vi "7.0.0_MAC Address reading.vi"(7 "Data in":T1, 8 "error in (no error)":errorcluster, 9 "AllControls In":T2, 10 "?":T3, 11 "Message Queue out":T4) -> (0 "error out":errorcluster, 1 "Flow":string, 2 "Data":T3, 3 "Message Queue Out":T4, 5 "Data out":T1)   [LabVIEW 2017]
uses:
  Depends/AMC/subVIs/TypeDefs/amc_Message Queue.ctl
  Depends/AMC/subVIs/TypeDefs/amc_Message.ctl
  Depends/Tools/Keyed Array/Tools_KeyedArray KeyedArray.ctl
  Ctrls/Data.ctl
  Ctrls/AllControls.ctl
  Ctrls/CSV_Data.ctl
  DIPC 692 Daemon API/typdef/destination.ctl
  DIPC 692 Daemon API/typdef/device_mode.ctl
  Ctrls/PathChoose.ctl
  DIPC 692 Daemon API/typdef/read_nvm_section.ctl
  DIPC 692 Daemon API/typdef/get_parameter.ctl
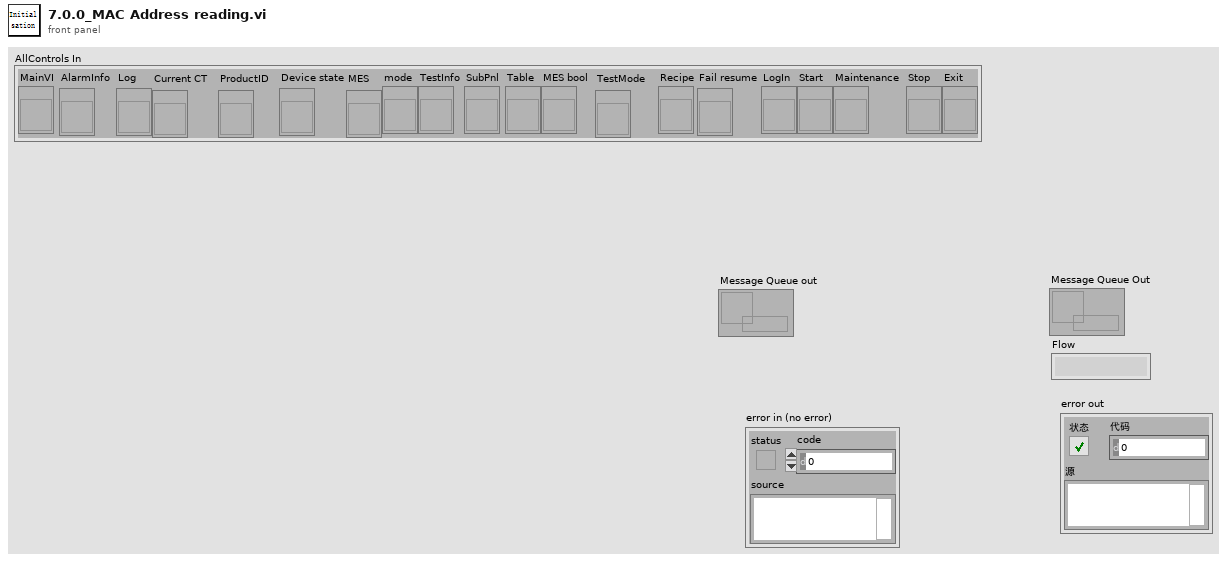
[diagram p1: front panel]
types:
  T1 = typedef "CSV_Data.ctl" = cluster{"Initialisation":cluster{"LMT - Connect UUT (con COM)":string, "LMT - Software Version (rrel)":string, "LMT - Write SKU file (wskuc)":string, "LMT - SKU file name":string, "Connect UUT DDM":string, "Read DDM EOL Timestamp - Mode":string, "Read DDM EOL Timestamp - Timestamp":string, "Read DDM EOL Timestamp - Rig ID":string, "Read DDM EOL Timestamp - Passmark ID":string, "Read DDM EOL Timestamp - Passmark Rev":string, "Software Version before flashing":string, "Read Hardware Serial":string, "UUT DDM SN":string, "Compare DDM SN with MES SN":string, "Backup PCBA Calibration EEPROM Response - CAL":string, "Flash Firmware Version":string, "Check SW Version":string, "Read DDM SW Version after flashing":string, "Set SKU Config":string, "Ready Status":string, "Set Device Mode to EOL":string, "DDM Parameter - Voltage":string, "DDM Parameter - Current":string, "DDM Parameter - Power":string, "DDM Parameter - Speed":string, "DDM Parameter - Pressure":string, "Tester Parameter - Voltage":string, "Tester Parameter - Current":string, "Tester Parameter - Power":string, "Tester Parameter - Ambient Pressure":string, "Tester Parameter - Ambient Temperature":string, "Calculated Parameter - DDM Pressure Corrected":string, "Calculated Parameter - DDM Real Power":string, "Calculated Parameter - Delta V":string}, "BEMF_Calibration":cluster{"Calibration Result - eol_cold_bemf_temp":string, "DDM Ambient Temp":string, "Restriction Plate Diameter":string, "Calibration Result - eol_bemf_mp_cold_coef_a":string, "Calibration Result - eol_bemf_mp_cold_coef_b":string, "Calibration Result - eol_bemf_mp_cold_coef_c":string, "Calibration Result - eol_bemf_lsi_cold_ref_coeffs":string, "Get - Calibration Result - eol_bemf_lsi_speed":string, "Get - Calibration Result - eol_bemf_lsi_integral_0":string, "Calibration Result - eol_bemf_lsi_integral_1":string, "Get - Calibration Result - eol_bemf_lsi_integral_2":string, "Get - Calibration Result - eol_cold_bemf":string, "Get - Calibration Result - eol_cold_bemf_fisf":string, "Finalise Calibration":string, "Compare -Calibration Result - eol_cold_bemf":string, "Compare -Calibration Result - eol_cold_bemf_fisf":string}, "ECO":cluster{"Reset Power Tune":string, "Reset BEMF FISF Calibration":string, "Restriction Plate Diameter":string, "ECO - Stabilisation Time":string, "ECO - DDM Parameter - Voltage":string, "ECO - DDM Parameter - Current":string, "ECO - DDM Parameter - Power":string, "ECO - DDM Parameter - Measured Power":string, "ECO - DDM Parameter - Speed":string, "ECO - DDM Parameter - Pressure":string, "ECO - Tester Parameter - Voltage":string, "ECO - Tester Parameter - Current":string, "ECO - Tester Parameter - Power":string, "ECO - Tester Parameter - Ambient Pressure":string, "ECO - Tester Parameter - Ambient Temperature":string, "ECO - Tester Parameter - Ambient Humidity":string, "ECO - Calculated Parameter - DDM Pressure Corrected":string, "ECO - Calculated Parameter - DDM Real Power":string, "ECO - Calculated Parameter - Delta V":string, "ECO - Calculated Parameter - Flowrate":string, "ECO - Calculated Parameter - Airwatt":string, "ECO - Formula":string, "PT ECO - Power Tune Mode Status":string}, "BOOST":cluster{"Restriction Plate Diameter":string, "BOOST - Stabilisation Time":string, "BOOST - DDM Parameter - Voltage":string, "BOOST - DDM Parameter - Current":string, "BOOST - DDM Parameter - Power":string, "BOOST - DDM Parameter - Measured Power":string, "BOOST - DDM Parameter - Speed":string, "BOOST - DDM Parameter - Pressure":string, "BOOST - Tester Parameter - Voltage":string, "BOOST - Tester Parameter - Current":string, "BOOST - Tester Parameter - Power":string, "BOOST - Tester Parameter - Ambient Pressure":string, "BOOST - Tester Parameter - Ambient Temperature":string, "BOOST - Tester Parameter - Ambient Humidity":string, "BOOST - Calculated Parameter - DDM Pressure Corrected":string, "BOOST - Calculated Parameter - DDM Real Power":string, "BOOST - Calculated Parameter - Delta V":string, "BOOST - Calculated Parameter - Flowrate":string, "BOOST - Calculated Parameter - Airwatt":string, "BOOST - Get AM Presence":string, "Air Muscle Turn Off Status":string, "BOOST - Air Muscle Calculated Parameter - Airwatt B":string, "BOOST - Air Muscle Calculate Airwatt Delta":string, "PT BOOST - Power Tune Mode Status":string, "Finalise Calibration":string, "ECO - Get AW Calibration value":string, "BOOST - Get AW Calibration value":string}, "MAX":cluster{"Restriction Plate Diameter":string, "MAX - Stabilisation Time":string, "Get Average Delta Tmag (LSIdelta_FISFdelta_LSItmag_FISFtmag_IIRtmag)":string, "Get Average Delta Tmag FISF":string, "MAX - DDM Parameter - Voltage":string, "MAX - DDM Parameter - Current":string, "MAX - DDM Parameter - Power":string, "MAX - DDM Parameter - Measured Power":string, "MAX - DDM Parameter - Speed":string, "MAX - DDM Parameter - Pressure":string, "MAX - Tester Parameter - Voltage":string, "MAX - Tester Parameter - Current":string, "MAX - Tester Parameter - Power":string, "MAX - Tester Parameter - Ambient Pressure":string, "MAX - Tester Parameter - Ambient Temperature":string, "MAX - Tester Parameter - Ambient Humidity":string, "MAX - Calculated Parameter - DDM Pressure Corrected":string, "MAX - Calculated Parameter - DDM Real Power":string, "MAX - Calculated Parameter - Delta V":string, "MAX - Calculated Parameter - Flowrate":string, "MAX - Calculated Parameter - Airwatt":string, "MAX_FISF_Check_Average_Delta_Tmag":string, "MAX - FISF - BEMF Finetune Result":string, "MAX tune - Delta P1":string, "MAX tune - Calculated Parameter - Airwatt":string, "Calculate Delta Airwatts - MAX finetune - Delta P2":string, "MAX finetune - DDM Parameter - Voltage":string, "MAX finetune - DDM Parameter - Current":string, "MAX finetune - DDM Parameter - Power":string, "MAX finetune - DDM Parameter - Measured Power":string, "MAX finetune - DDM Parameter - Speed":string, "MAX finetune - DDM Parameter - Pressure":string, "MAX finetune - Tester Parameter - Voltage":string, "MAX finetune - Tester Parameter - Current":string, "MAX finetune - Tester Parameter - Power":string, "MAX finetune - Tester Parameter - Ambient Pressure":string, "MAX finetune - Tester Parameter - Ambient Temperature":string, "MAX finetune - Tester Parameter - Ambient Humidity":string, "MAX finetune - Calculated Parameter - DDM Pressure Corrected":string, "MAX finetune - Calculated Parameter - DDM Real Power":string, "MAX finetune - Calculated Parameter - Delta V":string, "MAX finetune - Calculated Parameter - Flowrate":string, "MAX finetune - Calculated Parameter - Airwatt":string, "Check Derate Result":string, "Delta Tmag FISF":string, "Get Hot BEMF Result":string, "Calculate delta Pressure":string, "Finalise Calibration":string, "Calculate & Check Delta BEMF":string, "Delta P Airwatts Value":string}, "LL":cluster{"DDM Ambient Temp":string, "Restriction Plate Diameter":string, "LL - DDM Parameter - Voltage":string, "LL - DDM Parameter - Current":string, "LL - DDM Parameter - Power":string, "LL - DDM Parameter - Measured Power":string, "LL - DDM Parameter - Speed":string, "LL - DDM Parameter - Pressure":string, "LL - Tester Parameter - Voltage":string, "LL - Tester Parameter - Current":string, "LL - Tester Parameter - Power":string, "LL - DDM Real Power":string, "LL - Calibrate Task Detect LL":string}, "HL":cluster{"HL - DDM Parameter - Voltage":string, "HL - DDM Parameter - Current":string, "HL - DDM Parameter - Power":string, "HL - DDM Parameter - Measured Power":string, "HL - DDM Parameter - Speed":string, "HL - DDM Parameter - Pressure":string, "HL - Tester Parameter - Voltage":string, "HL - Tester Parameter - Current":string, "HL - Tester Parameter - Power":string, "HL - DDM Real Power":string, "HL - Calibrate Task Detect HL":string}, "LH":cluster{"Restriction Plate Diameter":string, "LH - DDM Parameter - Voltage":string, "LH - DDM Parameter - Current":string, "LH - DDM Parameter - Power":string, "LH - DDM Parameter - Measured Power":string, "LH - DDM Parameter - Speed":string, "LH - DDM Parameter - Pressure":string, "LH - Tester Parameter - Voltage":string, "LH - Tester Parameter - Current":string, "LH - Tester Parameter - Power":string, "LH - DDM Real Power":string, "LH - Calibrate Task Detect LH":string}, "HH":cluster{"HH - DDM Parameter - Voltage":string, "HH - DDM Parameter - Current":string, "HH - DDM Parameter - Power":string, "HH - DDM Parameter - Measured Power":string, "HH - DDM Parameter - Speed":string, "HH - DDM Parameter - Pressure":string, "HH - Tester Parameter - Voltage":string, "HH - Tester Parameter - Current":string, "HH - Tester Parameter - Power":string, "HH - DDM Real Power":string, "HH - Calibrate Task Detect HH":string}, "Inlet Blockage Calibration":cluster{"Inlet Blockage Calibration - DDM Parameter - Voltage":string, "Inlet Blockage Calibration - DDM Parameter - Current":string, "Inlet Blockage Calibration - DDM Parameter - Power":string, "Inlet Blockage Calibration - DDM Parameter - Measured Power":string, "Inlet Blockage Calibration - DDM Parameter - Speed":string, "Inlet Blockage Calibration - DDM Parameter - Pressure":string, "Inlet Blockage Calibration - Tester Parameter - Voltage":string, "Inlet Blockage Calibration - Tester Parameter - Current":string, "Inlet Blockage Calibration - Tester Parameter - Power":string, "Inlet Blockage Calibration - DDM Real Power":string, "Calibration Inlet Blockage_E":string, "Finalise Calibration":string, "Get Task Detect LL":string, "Get Task Detect HL":string, "Get Task Detect LH":string, "Get Task Detect HH":string, "Calibration Inlet Blockage":string, "Calibration eol cold bemf temp":string}, "GOOD":cluster{"GOOD UNIT - Clear EEPROM Error Log":string, "GOOD UNIT - Write Product Timestamp - Mode":string, "GOOD UNIT - Write Product Timestamp - Timestamp":string, "GOOD UNIT - Write Product Timestamp - Rig ID":string, "GOOD UNIT - Write Product Timestamp - Passmark ID":string, "GOOD UNIT - Write Product Timestamp - Passmark Rev":string, "GOOD UNIT - Set Device Mode to PROD":string, "GOOD UNIT - Backup PCBA Calibration EEPROM Response":string, "GOOD UNIT - Check Security Bit":string, "GOOD UNIT - Set Calibration Lock":string, "GOOD UNIT - Get_Calibration_Lock":string, "GOOD UNIT - Disconnect UUT":string}, "NG":cluster{"NG UNIT - Read NVM Error":string, "NG UNIT - Set Device Mode to FCT":string, "NG UNIT - Backup PCBA Calibration EEPROM Response - CAL":string, "NG UNIT - Backup PCBA Calibration EEPROM Response - ERROR":string, "NG UNIT - Backup PCBA Calibration EEPROM Response - USAGE":string, "NG UNIT - Disconnect UUT":string}, "SN":string, "Table":string[][], "Count":cluster{"Total":i32, "OK":i32, "NG":i32, "Yield":dbl}, "Start Time":timestamp, "daemon reference":refnum<k5>, "CT":dbl, "Config":string[][], "OK/NG":bool, "Station ID":string, "MES DDM SN":string, "MES PCBA SN":string, "Retest":string, "Lux":string, "Initialisation_Status":cluster{"LMT - Connect UUT (con COM)":string, "LMT - Software Version (rrel)":string, "LMT - Write SKU file (wskuc)":string, "LMT - SKU file name":string, "Connect UUT DDM":string, "Read DDM EOL Timestamp - Mode":string, "Read DDM EOL Timestamp - Timestamp":string, "Read DDM EOL Timestamp - Rig ID":string, "Read DDM EOL Timestamp - Passmark ID":string, "Read DDM EOL Timestamp - Passmark Rev":string, "Software Version before flashing":string, "Read Hardware Serial":string, "UUT DDM SN":string, "Compare DDM SN with MES SN":string, "Backup PCBA Calibration EEPROM Response - CAL":string, "Flash Firmware Version":string, "Check SW Version":string, "Read DDM SW Version after flashing":string, "Set SKU Config":string, "Ready Status":string, "Set Device Mode to EOL":string, "DDM Parameter - Voltage":string, "DDM Parameter - Current":string, "DDM Parameter - Power":string, "DDM Parameter - Speed":string, "DDM Parameter - Pressure":string, "Tester Parameter - Voltage":string, "Tester Parameter - Current":string, "Tester Parameter - Power":string, "Tester Parameter - Ambient Pressure":string, "Tester Parameter - Ambient Temperature":string, "Calculated Parameter - DDM Pressure Corrected":string, "Calculated Parameter - DDM Real Power":string, "Calculated Parameter - Delta V":string}, "BEMF_Calibration_Status":cluster{"Calibration Result - eol_cold_bemf_temp":string, "DDM Ambient Temp":string, "Restriction Plate Diameter":string, "Calibration Result - eol_bemf_mp_cold_coef_a":string, "Calibration Result - eol_bemf_mp_cold_coef_b":string, "Calibration Result - eol_bemf_mp_cold_coef_c":string, "Calibration Result - eol_bemf_lsi_cold_ref_coeffs":string, "Get - Calibration Result - eol_bemf_lsi_speed":string, "Get - Calibration Result - eol_bemf_lsi_integral_0":string, "Calibration Result - eol_bemf_lsi_integral_1":string, "Get - Calibration Result - eol_bemf_lsi_integral_2":string, "Get - Calibration Result - eol_cold_bemf":string, "Get - Calibration Result - eol_cold_bemf_fisf":string, "Finalise Calibration":string, "Compare -Calibration Result - eol_cold_bemf":string, "Compare -Calibration Result - eol_cold_bemf_fisf":string}, "ECO_Status":cluster{"Reset Power Tune":string, "Reset BEMF FISF Calibration":string, "Restriction Plate Diameter":string, "ECO - Stabilisation Time":string, "ECO - DDM Parameter - Voltage":string, "ECO - DDM Parameter - Current":string, "ECO - DDM Parameter - Power":string, "ECO - DDM Parameter - Measured Power":string, "ECO - DDM Parameter - Speed":string, "ECO - DDM Parameter - Pressure":string, "ECO - Tester Parameter - Voltage":string, "ECO - Tester Parameter - Current":string, "ECO - Tester Parameter - Power":string, "ECO - Tester Parameter - Ambient Pressure":string, "ECO - Tester Parameter - Ambient Temperature":string, "ECO - Tester Parameter - Ambient Humidity":string, "ECO - Calculated Parameter - DDM Pressure Corrected":string, "ECO - Calculated Parameter - DDM Real Power":string, "ECO - Calculated Parameter - Delta V":string, "ECO - Calculated Parameter - Flowrate":string, "ECO - Calculated Parameter - Airwatt":string, "ECO - Formula":string, "PT ECO - Power Tune Mode Status":string}, "BOOST_Status":cluster{"Restriction Plate Diameter":string, "BOOST - Stabilisation Time":string, "BOOST - DDM Parameter - Voltage":string, "BOOST - DDM Parameter - Current":string, "BOOST - DDM Parameter - Power":string, "BOOST - DDM Parameter - Measured Power":string, "BOOST - DDM Parameter - Speed":string, "BOOST - DDM Parameter - Pressure":string, "BOOST - Tester Parameter - Voltage":string, "BOOST - Tester Parameter - Current":string, "BOOST - Tester Parameter - Power":string, "BOOST - Tester Parameter - Ambient Pressure":string, "BOOST - Tester Parameter - Ambient Temperature":string, "BOOST - Tester Parameter - Ambient Humidity":string, "BOOST - Calculated Parameter - DDM Pressure Corrected":string, "BOOST - Calculated Parameter - DDM Real Power":string, "BOOST - Calculated Parameter - Delta V":string, "BOOST - Calculated Parameter - Flowrate":string, "BOOST - Calculated Parameter - Airwatt":string, "BOOST - Get AM Presence":string, "Air Muscle Turn Off Status":string, "BOOST - Air Muscle Calculated Parameter - Airwatt B":string, "BOOST - Air Muscle Calculate Airwatt Delta":string, "PT BOOST - Power Tune Mode Status":string, "Finalise Calibration":string, "ECO - Get AW Calibration value":string, "BOOST - Get AW Calibration value":string}, "MAX_Status":cluster{"Restriction Plate Diameter":string, "MAX - Stabilisation Time":string, "Get Average Delta Tmag (LSIdelta_FISFdelta_LSItmag_FISFtmag_IIRtmag)":string, "Get Average Delta Tmag FISF":string, "MAX - DDM Parameter - Voltage":string, "MAX - DDM Parameter - Current":string, "MAX - DDM Parameter - Power":string, "MAX - DDM Parameter - Measured Power":string, "MAX - DDM Parameter - Speed":string, "MAX - DDM Parameter - Pressure":string, "MAX - Tester Parameter - Voltage":string, "MAX - Tester Parameter - Current":string, "MAX - Tester Parameter - Power":string, "MAX - Tester Parameter - Ambient Pressure":string, "MAX - Tester Parameter - Ambient Temperature":string, "MAX - Tester Parameter - Ambient Humidity":string, "MAX - Calculated Parameter - DDM Pressure Corrected":string, "MAX - Calculated Parameter - DDM Real Power":string, "MAX - Calculated Parameter - Delta V":string, "MAX - Calculated Parameter - Flowrate":string, "MAX - Calculated Parameter - Airwatt":string, "MAX_FISF_Check_Average_Delta_Tmag":string, "MAX - FISF - BEMF Finetune Result":string, "MAX tune - Delta P1":string, "MAX tune - Calculated Parameter - Airwatt":string, "Calculate Delta Airwatts - MAX finetune - Delta P2":string, "MAX finetune - DDM Parameter - Voltage":string, "MAX finetune - DDM Parameter - Current":string, "MAX finetune - DDM Parameter - Power":string, "MAX finetune - DDM Parameter - Measured Power":string, "MAX finetune - DDM Parameter - Speed":string, "MAX finetune - DDM Parameter - Pressure":string, "MAX finetune - Tester Parameter - Voltage":string, "MAX finetune - Tester Parameter - Current":string, "MAX finetune - Tester Parameter - Power":string, "MAX finetune - Tester Parameter - Ambient Pressure":string, "MAX finetune - Tester Parameter - Ambient Temperature":string, "MAX finetune - Tester Parameter - Ambient Humidity":string, "MAX finetune - Calculated Parameter - DDM Pressure Corrected":string, "MAX finetune - Calculated Parameter - DDM Real Power":string, "MAX finetune - Calculated Parameter - Delta V":string, "MAX finetune - Calculated Parameter - Flowrate":string, "MAX finetune - Calculated Parameter - Airwatt":string, "Check Derate Result":string, "Delta Tmag FISF":string, "Get Hot BEMF Result":string, "Calculate delta Pressure":string, "Finalise Calibration":string, "Calculate & Check Delta BEMF":string, "Delta P Airwatts Value":string}, "LL_Status":cluster{"DDM Ambient Temp":string, "Restriction Plate Diameter":string, "LL - DDM Parameter - Voltage":string, "LL - DDM Parameter - Current":string, "LL - DDM Parameter - Power":string, "LL - DDM Parameter - Measured Power":string, "LL - DDM Parameter - Speed":string, "LL - DDM Parameter - Pressure":string, "LL - Tester Parameter - Voltage":string, "LL - Tester Parameter - Current":string, "LL - Tester Parameter - Power":string, "LL - DDM Real Power":string, "LL - Calibrate Task Detect LL":string}, "HL_Status":cluster{"HL - DDM Parameter - Voltage":string, "HL - DDM Parameter - Current":string, "HL - DDM Parameter - Power":string, "HL - DDM Parameter - Measured Power":string, "HL - DDM Parameter - Speed":string, "HL - DDM Parameter - Pressure":string, "HL - Tester Parameter - Voltage":string, "HL - Tester Parameter - Current":string, "HL - Tester Parameter - Power":string, "HL - DDM Real Power":string, "HL - Calibrate Task Detect HL":string}, "LH_Status":cluster{"Restriction Plate Diameter":string, "LH - DDM Parameter - Voltage":string, "LH - DDM Parameter - Current":string, "LH - DDM Parameter - Power":string, "LH - DDM Parameter - Measured Power":string, "LH - DDM Parameter - Speed":string, "LH - DDM Parameter - Pressure":string, "LH - Tester Parameter - Voltage":string, "LH - Tester Parameter - Current":string, "LH - Tester Parameter - Power":string, "LH - DDM Real Power":string, "LH - Calibrate Task Detect LH":string}, "HH_Status":cluster{"HH - DDM Parameter - Voltage":string, "HH - DDM Parameter - Current":string, "HH - DDM Parameter - Power":string, "HH - DDM Parameter - Measured Power":string, "HH - DDM Parameter - Speed":string, "HH - DDM Parameter - Pressure":string, "HH - Tester Parameter - Voltage":string, "HH - Tester Parameter - Current":string, "HH - Tester Parameter - Power":string, "HH - DDM Real Power":string, "HH - Calibrate Task Detect HH":string}, "Inlet Blockage Calibration_Status":cluster{"Inlet Blockage Calibration - DDM Parameter - Voltage":string, "Inlet Blockage Calibration - DDM Parameter - Current":string, "Inlet Blockage Calibration - DDM Parameter - Power":string, "Inlet Blockage Calibration - DDM Parameter - Measured Power":string, "Inlet Blockage Calibration - DDM Parameter - Speed":string, "Inlet Blockage Calibration - DDM Parameter - Pressure":string, "Inlet Blockage Calibration - Tester Parameter - Voltage":string, "Inlet Blockage Calibration - Tester Parameter - Current":string, "Inlet Blockage Calibration - Tester Parameter - Power":string, "Inlet Blockage Calibration - DDM Real Power":string, "Calibration Inlet Blockage_E":string, "Finalise Calibration":string, "Get Task Detect LL":string, "Get Task Detect HL":string, "Get Task Detect LH":string, "Get Task Detect HH":string, "Calibration Inlet Blockage":string, "Calibration eol cold bemf temp":string}, "GOOD_Status":cluster{"GOOD UNIT - Clear EEPROM Error Log":string, "GOOD UNIT - Write Product Timestamp - Mode":string, "GOOD UNIT - Write Product Timestamp - Timestamp":string, "GOOD UNIT - Write Product Timestamp - Rig ID":string, "GOOD UNIT - Write Product Timestamp - Passmark ID":string, "GOOD UNIT - Write Product Timestamp - Passmark Rev":string, "GOOD UNIT - Set Device Mode to PROD":string, "GOOD UNIT - Backup PCBA Calibration EEPROM Response":string, "GOOD UNIT - Check Security Bit":string, "GOOD UNIT - Set Calibration Lock":string, "GOOD UNIT - Get_Calibration_Lock":string, "GOOD UNIT - Disconnect UUT":string}, "NG_Status":cluster{"NG UNIT - Read NVM Error":string, "NG UNIT - Set Device Mode to FCT":string, "NG UNIT - Backup PCBA Calibration EEPROM Response - CAL":string, "NG UNIT - Backup PCBA Calibration EEPROM Response - ERROR":string, "NG UNIT - Backup PCBA Calibration EEPROM Response - USAGE":string, "NG UNIT - Disconnect UUT":string}, "SKU":string, "Plate_Diameter":string, "Alarm":string}
  T2 = typedef "AllControls.ctl" = cluster{"MainVI":refnum<vi>, "AlarmInfo":refnum<vi>, "Log":refnum<vi>, "Current CT":refnum<vi>, "ProductID":refnum<vi>, "Device state":refnum<vi>, "MES":refnum<vi>, "mode":refnum<vi>, "TestInfo":refnum<vi>, "SubPnl":refnum<vi>, "Table":refnum<vi>, "MES bool":refnum<vi>, "TestMode":refnum<vi>, "Recipe":refnum<vi>, "Fail resume":refnum<vi>, "LogIn":refnum<vi>, "Start":refnum<vi>, "Maintenance":refnum<vi>, "Stop":refnum<vi>, "Exit":refnum<vi>}
  T3 = typedef "Data.ctl" = cluster{"Initialisation":cluster{"DDM_Parameter":dbl[], "DDM_Parameter_status":bool[], "Get_Tester_Parameter":dbl[], "Get_Tester_Parameter_status":bool[], "Cal_Tester_Parameter":dbl[], "Cal_Tester_Parameter_status":bool[], "sw_version_before_status":bool, "sw_version_after_status":bool, "Set_SKU_Config_With_LMT_status":bool, "FCT_timestamp_status":bool, "LMT_Connect_to_UUT_status":bool}, "BEMF_Calibration":cluster{"Read_ambient_temperature":dbl, "Calibration_Vaule":dbl[], "Calibration_Vaule _B":dbl[], "Calibration_Vaule_status":bool[], "Calibration_Vaule_B_status":bool[]}, "ECO":cluster{"DDM_Parameter":dbl[], "DDM_Parameter_status":bool[], "Get_Tester_Parameter":dbl[], "Get_Tester_Parameter_status":bool[], "Cal_Tester_Parameter":dbl[], "Cal_Tester_Parameter_status":bool[], "DDM_Parameter_after_power_tune":dbl[], "Get_Tester_Parameter_after_power_tune":dbl[], "Cal_Tester_Parameter_after_power_tune":dbl[], "Cal_Tester_Parameter_after_power_tune_status":bool[], "Delta_P":dbl}, "BOOST":cluster{"DDM_Parameter":dbl[], "DDM_Parameter_status":bool[], "Get_Tester_Parameter":dbl[], "Get_Tester_Parameter_status":bool[], "Cal_Tester_Parameter":dbl[], "Cal_Tester_Parameter_status":bool[], "DDM_Parameter_after_power_tune":dbl[], "Get_Tester_Parameter_after_power_tune":dbl[], "Cal_Tester_Parameter_after_power_tune":dbl[], "Cal_Tester_Parameter_after_power_tune_status":bool[], "airwatts_am_off":dbl, "AW_Delta_(AM_on_and_off)":dbl, "AW_Delta_(AM_on_and_off)_Status":bool, "Delta_P":dbl}, "MAX":cluster{"Average_Tmag_Data":cluster{"LSI Delta in degC":dbl, "FISF Delta in degc":dbl, "LSI Tmag in degC":dbl, "Fisf Tmag in degC":dbl, "IIR Tmag in degC":dbl}, "DDM_Parameter":dbl[], "DDM_Parameter_status":bool[], "Get_Tester_Parameter":dbl[], "Get_Tester_Parameter_status":bool[], "Cal_Tester_Parameter":dbl[], "BEMF_Finetune":cluster{"eol_bemf_mp_cold_coef_c":dbl, "eol_cold_bemf_fisf_offset":dbl}, "AW_Tune":cluster{"delta_P1":dbl, "delta_P_Setting":dbl}, "DDM_Parameter_after_Airwatts_Tune":dbl[], "Get_Tester_Parameter_after_Airwatts_Tune":dbl[], "Cal_Tester_Parameter_after_Airwatts_Tune":dbl[], "DDM_Parameter_after_Airwatts_Finetune":dbl[], "Get_Tester_Parameter_after_Airwatts_Finetune":dbl[], "Cal_Tester_Parameter_after_Airwatts_Finetune":dbl[], "AW_Finetune":cluster{"delta_P2":dbl, "delta_P_Setting":dbl}, "Delta_Tmag_after_tune":cluster{"LSI Delta in degC":dbl, "FISF Delta in degc":dbl, "LSI Tmag in degC":dbl, "Fisf Tmag in degC":dbl, "IIR Tmag in degC":dbl}, "Hot Bemf in mV":dbl, "DDM_Pressure":dbl, "Delta_Pressure":dbl, " Cold Bemf in mV":dbl, " delta Bemf":dbl, " delta p":dbl, "Delta_Pressure_status":bool, " delta Bemf_status":bool, "LSI Delta in degC_status":bool, "FISF Delta in degc_status":bool, "Max_check_derate_status_status":bool, "Average_All_data":dbl[][], "Average_Tmag_Data_status":bool[], "Average_Tmag_Data_after_tune_status":bool[], "Cal_Tester_Parameter_status":bool[], "Cal_Tester_Parameter_status_after_Airwatts_Tune":bool[], "Cal_Tester_Parameter_status_after_Airwatts_FineTune":bool[]}, "Task_Detect_Calib":cluster{"LL":cluster{"DDM_Parameter":dbl[], "DDM_Parameter_status":bool[], "Get_Tester_Parameter":dbl[], "Get_Tester_Parameter_status":bool[], "Set_task_detect_A":dbl, "Set_task_detect_A_Status":bool}, "HL":cluster{"DDM_Parameter":dbl[], "DDM_Parameter_status":bool[], "Get_Tester_Parameter":dbl[], "Get_Tester_Parameter_status":bool[], "Set_task_detect_B":dbl, "Set_task_detect_B_Status":bool}, "LH":cluster{"DDM_Parameter":dbl[], "DDM_Parameter_status":bool[], "Get_Tester_Parameter":dbl[], "Get_Tester_Parameter_status":bool[], "Set_task_detect_C":dbl, "Set_task_detect_C_Status":bool}, "HH":cluster{"DDM_Parameter":dbl[], "DDM_Parameter_status":bool[], "Get_Tester_Parameter":dbl[], "Get_Tester_Parameter_status":bool[], "Set_task_detect_D":dbl, "Read_and_check_calibration_Status":bool[], "Set_task_detect_D_Status":bool}, "Get_eol_inlet_blockage_E":dbl, "Calib_vaule":cluster{"Get_task_detect_LL":dbl, "Get_task_detect_HL":dbl, "Get_task_detect_LH":dbl, "Get_task_detect_HH":dbl, "eol_inlet_blockage":dbl, "eol_code_bemf_temp":dbl}, "calibrated temp":dbl, "Inlet_Blockage_Calibration":cluster{"DDM_Parameter":dbl[], "DDM_Parameter_status":bool[], "Get_Tester_Parameter":dbl[], "Get_Tester_Parameter_status":bool[]}, "Get_eol_inlet_blockage_E_Status":bool}, "good":cluster{"Write_Product_TS":cluster{"TIMESTAMP":i64, "RIG_ID":i64, "PASSMARK_ID":i64, "PASSMARK_REV":i64}, "Read_Product_TS":cluster{"TIMESTAMP":i64, "RIG_ID":i64, "PASSMARK_ID":i64, "PASSMARK_REV":i64}, "Good_Check_Secuity_Bit_Stauts":bool}}
  T4 = typedef "amc_Message Queue.ctl" = refnum<queue>
  T5 = cluster{"Brush_ADC.bat":string, "Get Release Version.bat":string, "Getting Software  Version.bat":string, "Pump_ADC.bat":string, "Starting  Pump Motor.bat":string, "Starting  Test Mode.bat":string, "Starting Brush Motor 1.bat":string, "Starting Brush Motor 2.bat":string, "Starting Brush Motor 3.bat":string, "Starting LED Test.bat":string, "Stopping  Brush Motor.bat":string, "Stopping  Pump Motor.bat":string, "Stopping  Test Mode.bat":string, "1":string, "2":string, "3":string, "4":string, "5":string, "6":string, "7":string, "8":string, "9":string, "10":string}
  T6 = typedef "destination.ctl" = string
  T7 = typedef "PathChoose.ctl" = enum16{"OperatorLog", "AutoRunLog", "AlmLog", "TestData", "AllTestData", "backup_nvm", "backup_before_flashing"}
  T8 = enum16{"open", "replace", "create", "open or create", "replace or create", "replace or create with confirmation"}
  T9 = typedef "read_nvm_section.ctl" = enum16{"CAL", "ERROR", "USAGE"}
  T10 = typedef "get_parameter.ctl" = string
  T11 = typedef "HD Config.ctl" = cluster{" PC":cluster{"PC Address":u8[], "PC Port":i32}, "FCO":cluster{"COM":refnum<visa-resource-name>, "Baudrate":u32}, "DC Power ":cluster{"COM":refnum<visa-resource-name>, "Baudrate":u32}, "PW3336":cluster{"COM":refnum<visa-resource-name>, "Baudrate":u32}, "Lefoo":cluster{"COM":refnum<visa-resource-name>, "Baudrate":u32}, "Tempt&Hum":cluster{"COM":refnum<visa-resource-name>, "Baudrate":u32}, "DIPC":cluster{"COM":refnum<visa-resource-name>}, "Daemon":cluster{"IP Address":string, "Port":u16, "Retry":u16}, "URAT":cluster{"COM":refnum<visa-resource-name>, "Baudrate":u32}, "Fail_resume_mode":bool, "GRR":bool}
  T12 = typedef "device_mode.ctl" = enum16{"FCT", "EOL", "PROD"}
  T13 = cluster{"TIMESTAMP":i64, "RIG_ID":i64, "PASSMARK_ID":i64, "PASSMARK_REV":i64}
  T14 = cluster{"TIMESTAMP":string, "RIG_ID":string, "PASSMARK_ID":string, "PASSMARK_REV":string}
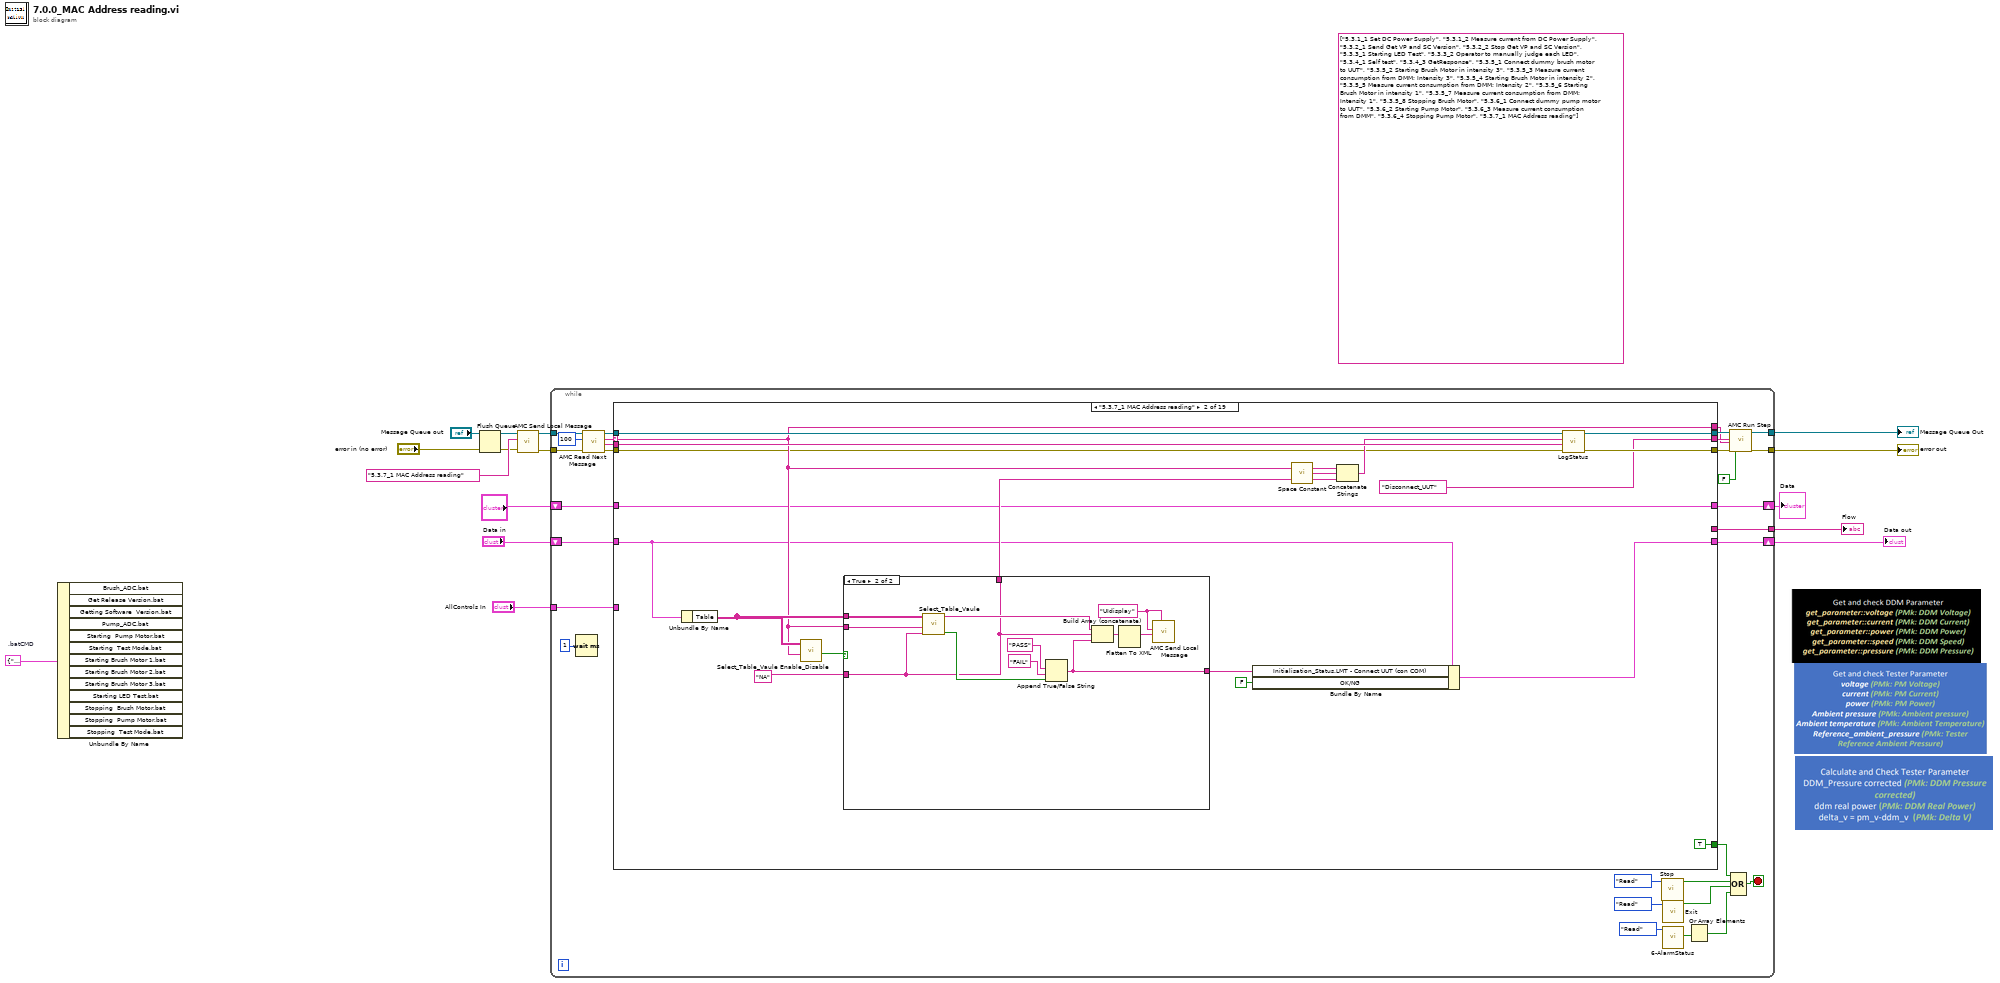
[diagram p0: block diagram]
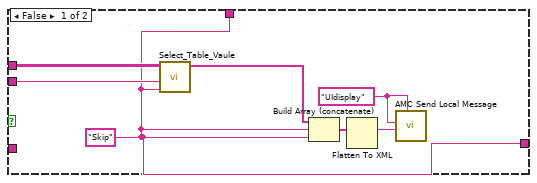
[diagram p3: hidden frame]
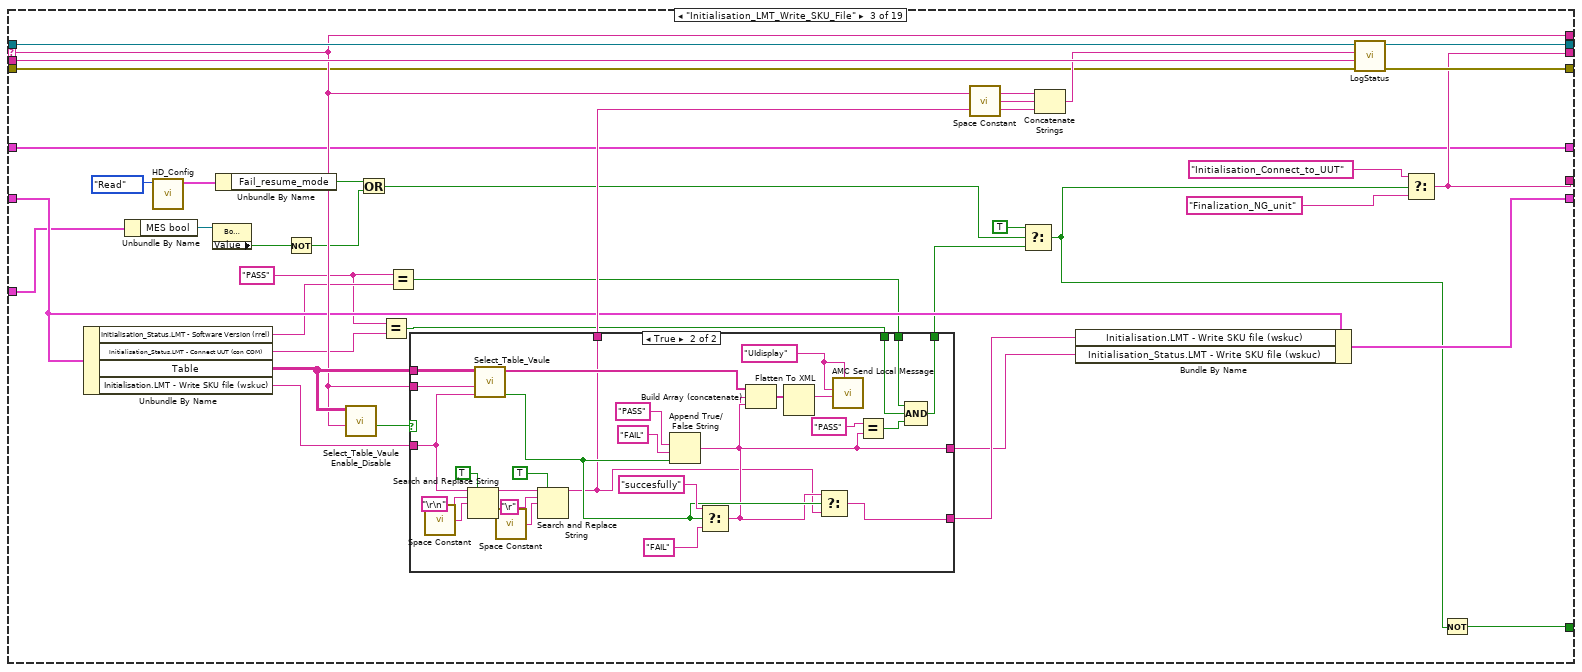
[diagram p4: hidden frame]
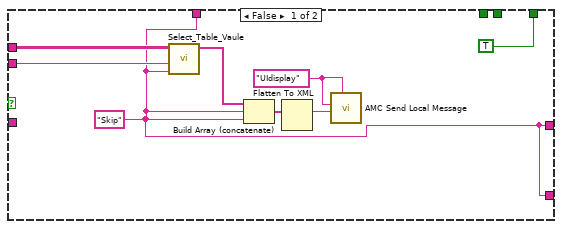
[diagram p5: hidden frame]
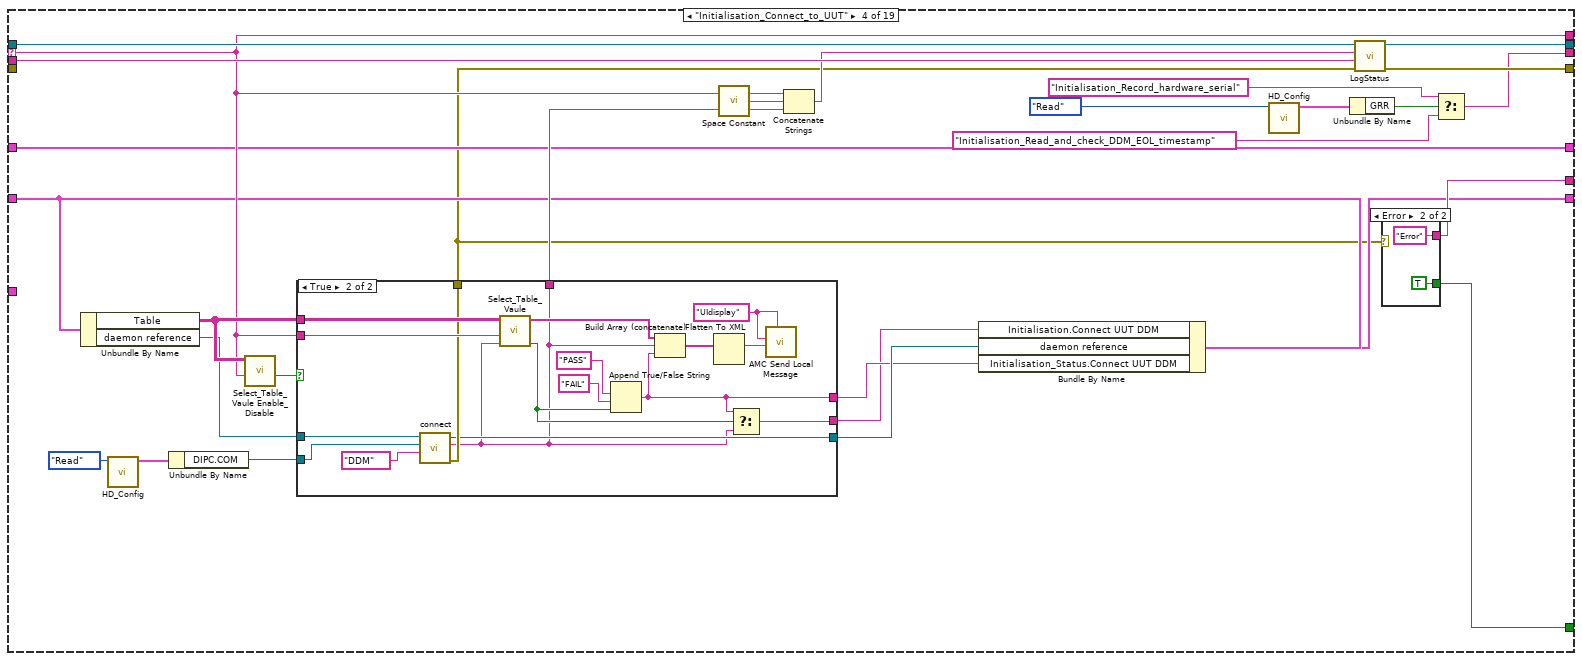
[diagram p6: hidden frame]
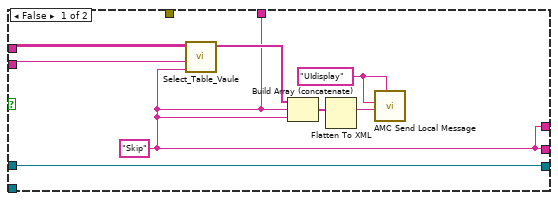
[diagram p8: hidden frame]
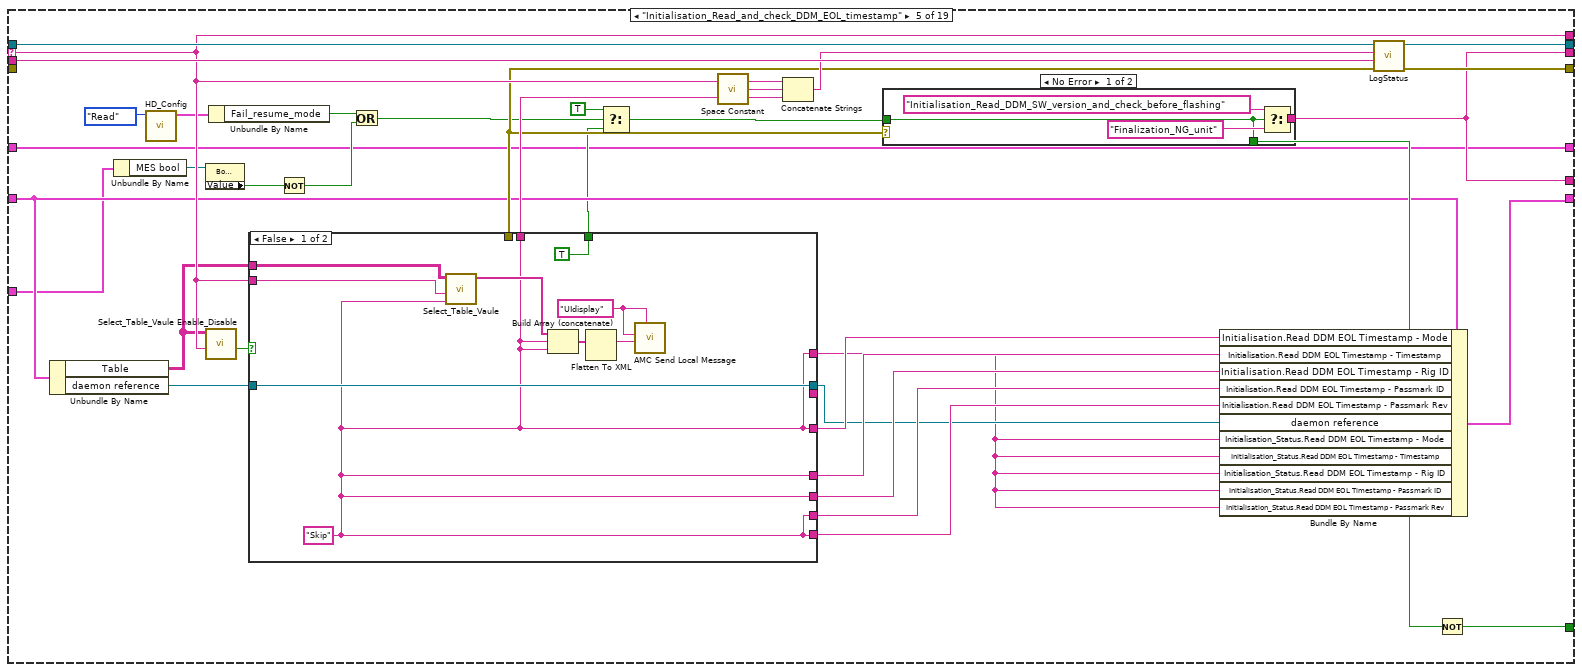
[diagram p9: hidden frame]
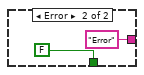
[diagram p10: hidden frame]
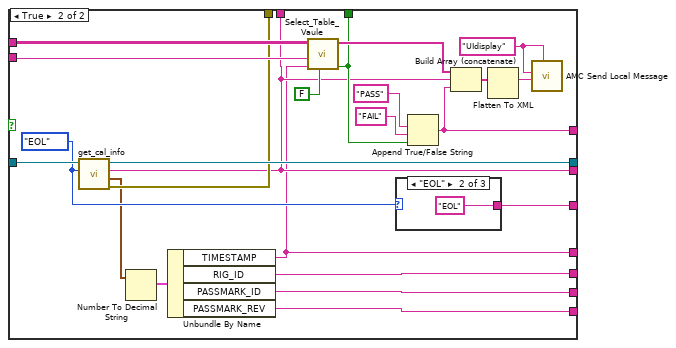
[diagram p11: hidden frame]
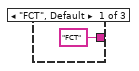
[diagram p12: hidden frame]
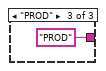
[diagram p13: hidden frame]
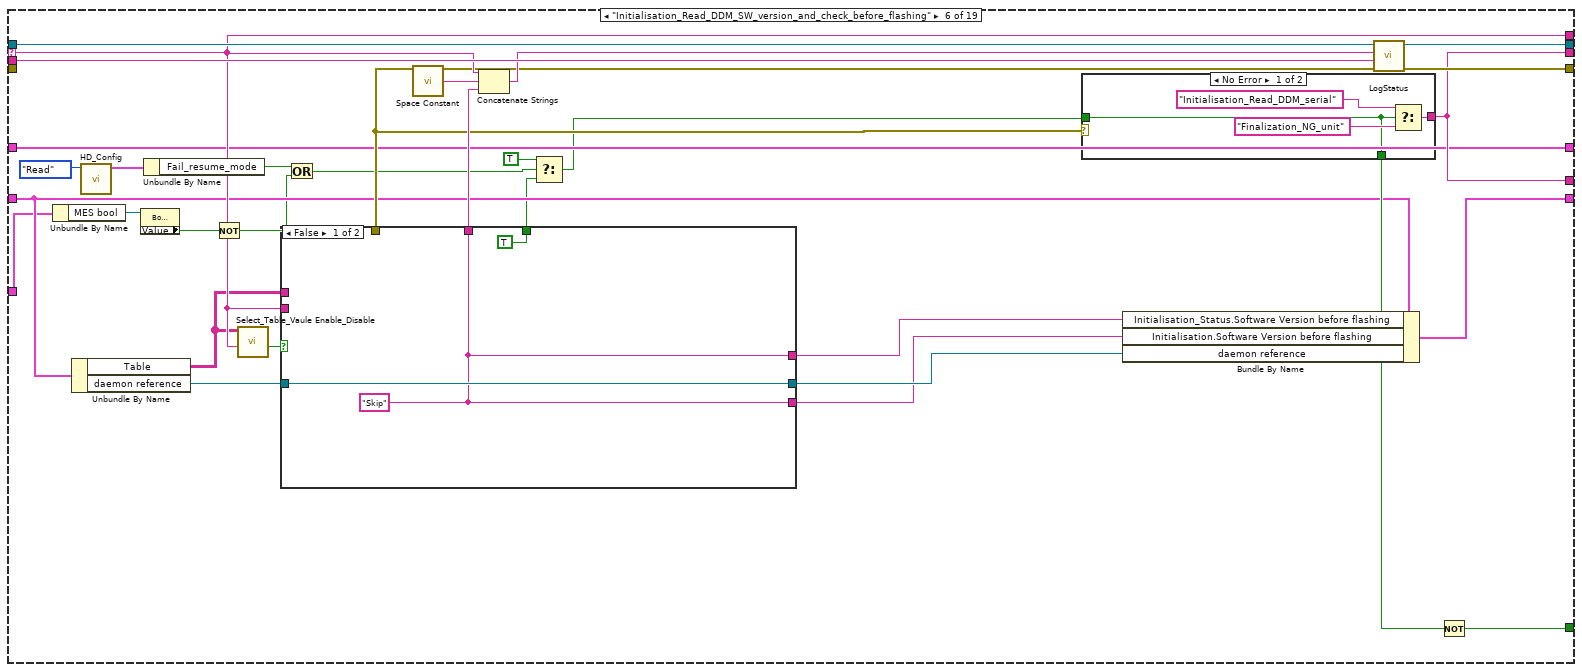
[diagram p14: hidden frame]
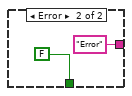
[diagram p15: hidden frame]
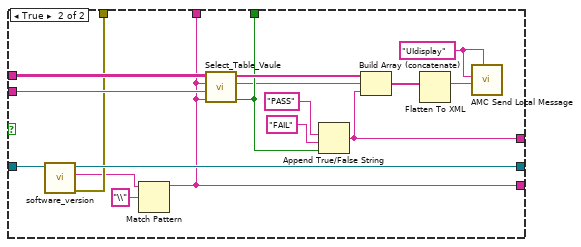
[diagram p16: hidden frame]
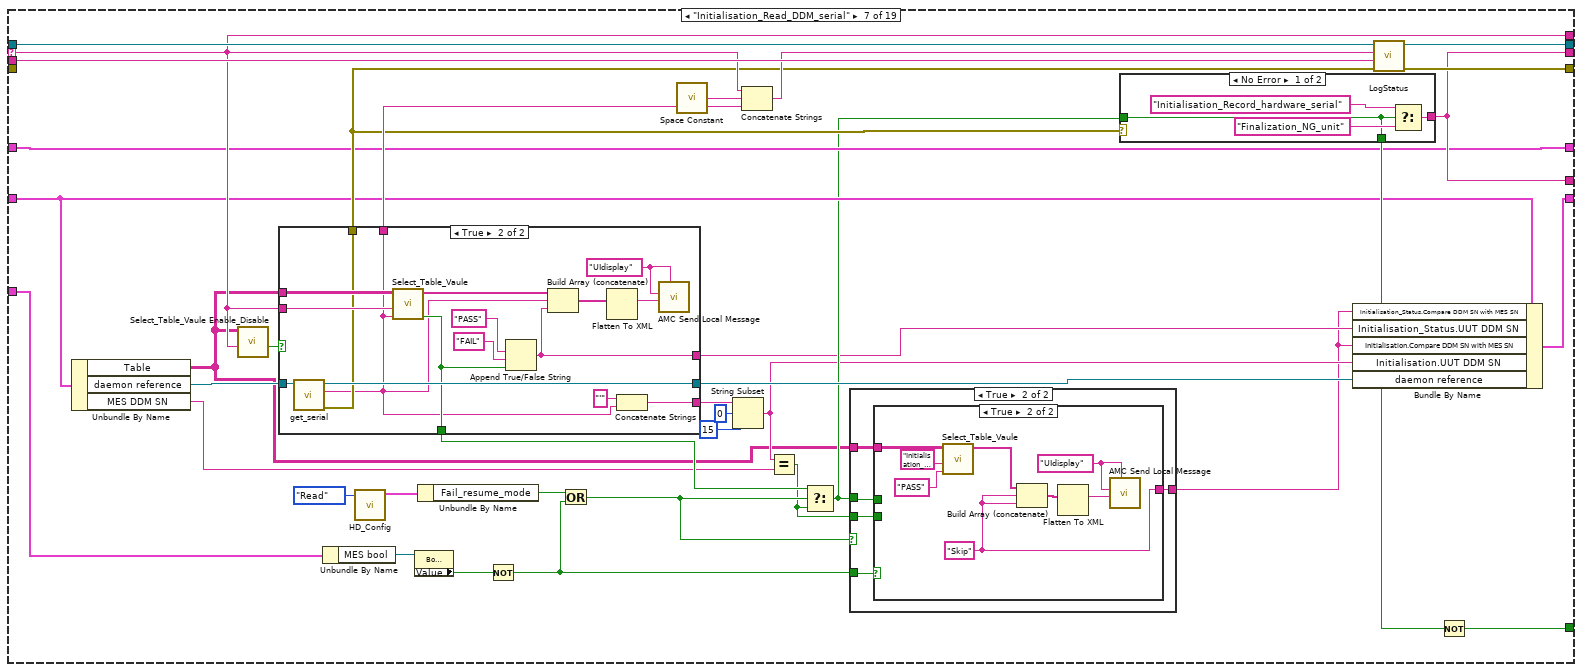
[diagram p17: hidden frame]
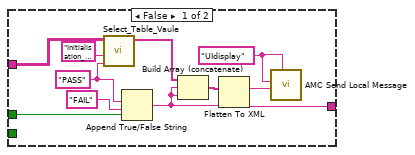
[diagram p18: hidden frame]
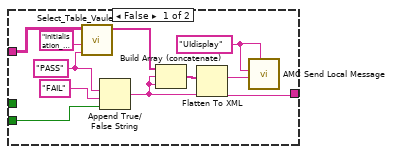
[diagram p19: hidden frame]
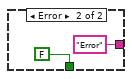
[diagram p20: hidden frame]
diagram:
  w1 = T5 {"Brush_ADC.bat"="Brush_ADC.bat", "Get Release Version.bat"="Get Release Version.bat", "Getting Software  Version.bat"="Getting Software  Version.bat", "Pump_ADC.bat"="Pump_ADC.bat", "Starting  Pump Motor.bat"="Starting  Pump Motor.bat", "Starting  Test Mode.bat"="Starting  Test Mode.bat", "Starting Brush Motor 1.bat"="Starting Brush Motor 1.bat", "Starting Brush Motor 2.bat"="Starting Brush Motor 2.bat", "Starting Brush Motor 3.bat"="Starting Brush Motor 3.bat", "Starting LED Test.bat"="Starting LED Test.bat", "Stopping  Brush Motor.bat"="Stopping  Brush Motor.bat", "Stopping  Pump Motor.bat"="Stopping  Pump Motor.bat", "Stopping  Test Mode.bat"="Stopping  Test Mode.bat", "1"="", "2"="", "3"="", "4"="", "5"="", "6"="", "7"="", "8"="", "9"="", "10"=""}  # .batCMD
  (unwired) string[] ["5.3.1_1 Set DC Power Supply", "5.3.1_2 Measure current from DC Power Supply", "5.3.2_1 Send Get VP and SC Version", "5.3.2_2 Stop Get VP and SC Version", "5.3.3_1 Starting LED Test", "5.3.3_2 Operator to manually judge each LED", "5.3.4_1 Self test", "5.3.4_3 GetResponse", "5.3.5_1 Connect dummy brush motor to UUT", "5.3.5_2 Starting Brush Motor in intensity 3", "5.3.5_3 Measure current consumption from DMM; Intensity 3", "5.3.5_4 Starting Brush Motor in intensity 2", "5.3.5_5 Measure current consumption from DMM; Intensity 2", "5.3.5_6 Starting Brush Motor in intensity 1", "5.3.5_7 Measure current consumption from DMM; Intensity 1", "5.3.5_8 Stopping Brush Motor", "5.3.6_1 Connect dummy pump motor to UUT", "5.3.6_2 Starting Pump Motor", "5.3.6_3 Measure current consumption from DMM", "5.3.6_4 Stopping Pump Motor", "5.3.7_1 MAC Address reading"] ("subarray")
  n1 = Unbundle By Name(w1) -> ()  [unwired: 13 out]
  n2 = Flush Queue(queue="Message Queue out") -> (queue out=w7:T4)  [unwired: 1 in, 2 out]
  n3 = call "AMC Send Local Message.vi"("error in (no error)"="error in (no error)", "Message Name"="5.3.7_1 MAC Address reading", "Message Queue in"=w7) -> ("error out"=w12:errorcluster, "Message Queue out"=w13:T4)  [unwired: 7 in]
  n4 = while {
    tunnel: w13 -> [w45]
    tunnel: [w41] -> w6
    tunnel: w12 -> [w39]
    tunnel: [w36] -> w5
    shift-right: [w32] -> w9
    shift-left: "?" -> [w33]
    tunnel: [w28] -> w8
    tunnel: "AllControls In" -> [w21]
    shift-right: [w19] -> w2
    shift-left: "Data in" -> [w20]
    stop <- w24 stop-if-true
    n5 = Wait (ms)(milliseconds to wait=u32 1 ("等待时间（毫秒）")) -> ()  [unwired: 1 out]
    n6 = call "AMC Read Next Message.vi"("error in (no error)"=w39, "timeout (1ms)"=100, "Message Queue in"=w45) -> ("error out"=w38:errorcluster, "Message Value"=w30:string, "Message Name"=w43:string, "Message Queue out"=w44:T4)  [unwired: 1 in, 4 out]
    n7 = case shown="\"5.3.7_1 MAC Address reading\"" w43 {
      selector: w43 -> [_ w61 w115 w177 w240 w311 w372 w455 w492 w542 w595 w700 w756 w820 w873 w935 w1027 w1112 w1172]
      tunnel: w44 -> [w49 w67 w121 w185 w247 w319 w380 w462 w499 w549 w601 w707 w762 w826 w879 w942 w1035 w1121 w1186]
      tunnel: [w49 w67 w121 w185 w247 w319 w380 w462 w499 w549 w601 w707 w762 w826 w879 w942 w1035 w1121 w1162] -> w42
      tunnel: w38 -> [w48 w60 w114 _ _ _ _ _ w498 _ _ _ _ _ _ _ w1034 w1120 w1189]
      tunnel: [w48 w66 w120 w184 w246 w318 w379 w461 w497 w548 w600 w706 w761 w825 w878 w941 w1033 w1119 w1187] -> w37
      tunnel: [_ TRUE ("GRR") w110 w171 w238 w308 w370 w451 _ w538 w585 w695 w751 w815 w863 w929 _ TRUE w1168] -> w25
      tunnel: w33 -> [w47 w56 w105 w168 w214 w302 w364 w446 w489 w516 w577 w679 w744 w797 w865 w922 w1017 w1100 w1173]
      tunnel: [w47 w56 w105 w168 w214 w302 w364 w446 w489 w516 w577 w679 w744 w797 w865 w921 w1016 w1116 w1184] -> w32
      tunnel: w30 -> [_ w65 w119 w183 w245 w317 w378 w460 w496 w547 w599 w705 w760 w824 w877 w940 w1032 w1118 w1188]
      tunnel: [_ w61 w115 w177 w240 w311 w372 w455 w492 w542 w595 w700 w756 w820 w873 w935 w1027 w1112 w1172] -> w29
      tunnel: [_ "Disconnect_UUT" w112 w161 w237 w309 w371 w441 w485 "Initialisation_Flash_SW_follow_SKU" w589 w696 w739 w816 w860 "Initialisation_Get_and_check_Tester_Parameter" "Initialisation_Calculate_and_check_tester_parameter" w1102 w1169] -> w31
      tunnel: [_ _ w112 w173 w237 w309 w371 w452 _ w537 w586 w696 w752 w816 w860 w930 _ w1102 w1169] -> w28
      tunnel: w21 -> [_ _ w100 _ w217 w295 w358 _ _ _ w584 w682 _ w802 _ _ _ w1085 _]
      tunnel: w20 -> [w46 w55 w104 w170 w232 w305 w367 w450 w482 w520 w581 w694 w748 w812 w864 w927 w1022 w1096 w1160]
      tunnel: [w46 w54 w103 w169 w234 w304 w366 w447 w482 w519 w580 w692 w745 w811 w867 w924 w1019 w1094 w1161] -> w19
      frame "假", Default {
      }
      frame "5.3.7_1 MAC Address reading" {
        n8 = Unbundle By Name(w55) -> ("Table"=w62:string[][])
        n9 = call "Select_Table_Vaule Enable_Disable.vi"("Action"=w61, "Table"=w62) -> ("Enable"=w58:bool)  [unwired: 8 in, 1 out]
        n10 = case shown="True" w58 {
          tunnel: [w68 w76] -> w59
          tunnel: w62 -> [w70 w79]
          tunnel: w61 -> [w69 w78]
          tunnel: "NA" ("elease version:") -> [_ w76]
          tunnel: [w68 w75] -> w53
          frame False {
            w74 = "UIdisplay" ("Process (\"\" - local)")
            w68 = "Skip" ("Action")
            n11 = call "Select_Table_Vaule.vi"("Vaule"=w68, "Action"=w69, "Table"=w70) -> ("vaule"=w71:string[])  [unwired: 7 in, 1 out]
            n12 = Build Array (concatenate)(w71, w68, w68) -> (w73:string[])
            n13 = Flatten To XML(anything=w73) -> (xml string=w72:string)
            n14 = call "AMC Send Local Message.vi"("Process (\"\" - local)"=w74, "Message Value"=w72, "Message Name"=w74) -> ()  [unwired: 7 in, 2 out]
          }
          frame True {
            w84 = "UIdisplay" ("Process (\"\" - local)")
            n15 = call "Select_Table_Vaule.vi"("Vaule"=w76, "Action"=w78, "Table"=w79) -> ("Result"=w77:bool, "vaule"=w85:string[])  [unwired: 7 in]
            n16 = Append True/False String(1:w77, 2:"FAIL" ("真字符串"), 3:"PASS" ("真字符串")) -> (0:w75:string)  [unwired: 1 in]
            n17 = Build Array (concatenate)(w85, w76, w75) -> (w83:string[])
            n18 = Flatten To XML(anything=w83) -> (xml string=w82:string)
            n19 = call "AMC Send Local Message.vi"("Process (\"\" - local)"=w84, "Message Value"=w82, "Message Name"=w84) -> ()  [unwired: 7 in, 2 out]
          }
        }
        n20 = Bundle By Name(cluster=w55, "Initialisation_Status.LMT - Connect UUT (con COM)"=w53, "OK/NG"=FALSE) -> (w54:T1)
        n21 = call <vilib>:"Space Constant.vi"() -> ("String"=w63:string)
        n22 = Concatenate Strings(w61, w63, w59) -> (w64:string)
        n23 = call "LogStatus.vi"("error in (no error)"=w60, "last message"=w65, "message"=w64) -> ("error  out"=w66:errorcluster)  [unwired: 8 in]
      }
      frame "Initialisation_LMT_Write_SKU_File" {
        w92 = "PASS" ("真字符串")
        n24 = Unbundle By Name(w104) -> ("Initialisation_Status.LMT - Software Version (rrel)"=w94:string, "Initialisation_Status.LMT - Connect UUT (con COM)"=w93:string, "Table"=w116:string[][], "Initialisation.LMT - Write SKU file (wskuc)"=w107:string)
        n25 = Unbundle By Name(w100) -> ("MES bool"=w99:refnum<vi>)
        n26 = call "HD_Config.vi"("Step"=enum16{"Initial", "Write", "Read"}."Read") -> ("HD Config out"=w101:T11)  [unwired: 9 in, 1 out]
        n27 = property class="Bool (严格)"(reference=w99) -> ("Value"=w97:bool)  [unwired: 1 in, 2 out]
        n28 = Unbundle By Name(w101) -> ("Fail_resume_mode"=w98:bool)
        n29 = Not(x=w97) -> (.not. x?=w96:bool)
        n30 = call "Select_Table_Vaule Enable_Disable.vi"("Action"=w115, "Table"=w116) -> ("Enable"=w108:bool)  [unwired: 8 in, 1 out]
        n31 = Or(x=w98, y=w96) -> (x .or. y?=w89:bool)
        n32 = Equal?(x=w92, y=w93) -> (x = y?=w87:bool)
        n33 = Equal?(x=w92, y=w94) -> (x = y?=w88:bool)
        n34 = case shown="True" w108 {
          tunnel: [w122 w136] -> w109
          tunnel: w116 -> [w124 w151]
          tunnel: w115 -> [w123 w150]
          tunnel: w107 -> [_ w141]
          tunnel: [w122 w135] -> w106
          tunnel: [w122 w139] -> w91
          tunnel: w88 -> [_ w133]
          tunnel: w87 -> [_ w132]
          tunnel: [TRUE w130] -> w86
          frame False {
            w128 = "UIdisplay" ("Process (\"\" - local)")
            w122 = "Skip" ("Action")
            n35 = call "Select_Table_Vaule.vi"("Vaule"=w122, "Action"=w123, "Table"=w124) -> ("vaule"=w125:string[])  [unwired: 7 in, 1 out]
            n36 = Build Array (concatenate)(w125, w122, w122) -> (w127:string[])
            n37 = Flatten To XML(anything=w127) -> (xml string=w126:string)
            n38 = call "AMC Send Local Message.vi"("Process (\"\" - local)"=w128, "Message Value"=w126, "Message Name"=w128) -> ()  [unwired: 7 in, 2 out]
          }
          frame True {
            w156 = "UIdisplay" ("Process (\"\" - local)")
            n39 = call <vilib>:"Space Constant.vi"() -> ("String"=w147:string)
            n40 = Search and Replace String(replace all?=TRUE ("replace all? (F)"), input string=w141, search string="\r\n", replace string=w147) -> (result string=w149:string)  [unwired: 4 in, 3 out]
            n41 = call "Select_Table_Vaule.vi"("Vaule"=w141, "Action"=w150, "Table"=w151) -> ("Result"=w138:bool, "vaule"=w157:string[])  [unwired: 7 in]
            n42 = call <vilib>:"Space Constant.vi"() -> ("String"=w148:string)
            n43 = Search and Replace String(replace all?=TRUE ("replace all? (F)"), input string=w149, search string="\r", replace string=w148) -> (result string=w136:string)  [unwired: 4 in, 3 out]
            n44 = Append True/False String(1:w138, 2:"FAIL" ("真字符串"), 3:"PASS" ("真字符串")) -> (0:w139:string)  [unwired: 1 in]
            n45 = Select(t="succesfully" ("真字符串"), s=w138, f="FAIL" ("真字符串")) -> (s? t:f=w137:string)
            n46 = Build Array (concatenate)(w157, w137, w139) -> (w155:string[])
            n47 = Flatten To XML(anything=w155) -> (xml string=w154:string)
            n48 = Select(t=w137, s=w138, f=w136) -> (s? t:f=w135:string)
            n49 = call "AMC Send Local Message.vi"("Process (\"\" - local)"=w156, "Message Value"=w154, "Message Name"=w156) -> ()  [unwired: 7 in, 2 out]
            n50 = Equal?(x="PASS" ("真字符串"), y=w139) -> (x = y?=w131:bool)
            n51 = Compound Arithmetic op=AND ("复合运算")(w133, w132, w131) -> (w130:bool)
          }
        }
        n52 = call <vilib>:"Space Constant.vi"() -> ("String"=w117:string)
        n53 = Select(t=TRUE, s=w89, f=w86) -> (s? t:f=w90:bool)
        n54 = Concatenate Strings(w115, w117, w109) -> (w118:string)
        n55 = Bundle By Name(cluster=w104, "Initialisation.LMT - Write SKU file (wskuc)"=w106, "Initialisation_Status.LMT - Write SKU file (wskuc)"=w91) -> (w103:T1)
        n56 = call "LogStatus.vi"("error in (no error)"=w114, "last message"=w119, "message"=w118) -> ("error  out"=w120:errorcluster)  [unwired: 8 in]
        n57 = Select(t="Initialisation_Connect_to_UUT", s=w90, f="Finalization_NG_unit") -> (s? t:f=w112:string)
        n58 = Not(x=w90) -> (.not. x?=w110:bool)
      }
      frame "Initialisation_Connect_to_UUT" {
        n59 = Unbundle By Name(w170) -> ("Table"=w178:string[][], "daemon reference"=w172:refnum<k5>)
        n60 = call "HD_Config.vi"("Step"=enum16{"Initial", "Write", "Read"}."Read") -> ("HD Config out"=w174:T11)  [unwired: 9 in, 1 out]
        n61 = Unbundle By Name(w174) -> ("DIPC.COM"=w182:refnum<visa-resource-name>)
        n62 = call "Select_Table_Vaule Enable_Disable.vi"("Action"=w177, "Table"=w178) -> ("Enable"=w176:bool)  [unwired: 8 in, 1 out]
        n63 = case shown="True" w176 {
          tunnel: w182 -> [_ w212]
          tunnel: [w188 w197] -> w179
          tunnel: w178 -> [w190 w205]
          tunnel: w177 -> [w189 w204]
          tunnel: [_ w203] -> w166
          tunnel: w172 -> [w195 w201]
          tunnel: [w188 w198] -> w159
          tunnel: [w195 w200] -> w167
          tunnel: [w188 w196] -> w158
          frame False {
            w191 = "UIdisplay" ("Process (\"\" - local)")
            w188 = "Skip" ("response")
            n64 = call "Select_Table_Vaule.vi"("Vaule"=w188, "Action"=w189, "Table"=w190) -> ("vaule"=w194:string[])  [unwired: 7 in, 1 out]
            n65 = Build Array (concatenate)(w194, w188, w188) -> (w192:string[])
            n66 = Flatten To XML(anything=w192) -> (xml string=w193:string)
            n67 = call "AMC Send Local Message.vi"("Process (\"\" - local)"=w191, "Message Value"=w193, "Message Name"=w191) -> ()  [unwired: 7 in, 2 out]
          }
          frame True {
            w210 = "UIdisplay" ("Process (\"\" - local)")
            n68 = call "connect.vi"("Target"=T6 "DDM", "physical connection"=w212, "daemon reference in"=w201) -> ("error out"=w203:errorcluster, "response"=w197:string, "daemon reference out"=w200:refnum<k5>)  [unwired: 4 in, 2 out]
            n69 = call "Select_Table_Vaule.vi"("Vaule"=w197, "Action"=w204, "Table"=w205) -> ("Result"=w199:bool, "vaule"=w211:string[])  [unwired: 7 in]
            n70 = Append True/False String(1:w199, 2:"FAIL" ("真字符串"), 3:"PASS" ("真字符串")) -> (0:w198:string)  [unwired: 1 in]
            n71 = Build Array (concatenate)(w211, w197, w198) -> (w209:string[])
            n72 = Flatten To XML(anything=w209) -> (xml string=w208:string)
            n73 = Select(t=w198, s=w199, f=w197) -> (s? t:f=w196:string)
            n74 = call "AMC Send Local Message.vi"("Process (\"\" - local)"=w210, "Message Value"=w208, "Message Name"=w210) -> ()  [unwired: 7 in, 2 out]
          }
        }
        n75 = call <vilib>:"Space Constant.vi"() -> ("String"=w180:string)
        n76 = Concatenate Strings(w177, w180, w179) -> (w181:string)
        n77 = Bundle By Name(cluster=w170, "Initialisation.Connect UUT DDM"=w158, "daemon reference"=w167, "Initialisation_Status.Connect UUT DDM"=w159) -> (w169:T1)
        n78 = call "HD_Config.vi"("Step"=enum16{"Initial", "Write", "Read"}."Read") -> ("HD Config out"=w165:T11)  [unwired: 9 in, 1 out]
        n79 = Unbundle By Name(w165) -> ("GRR"=w163:bool)
        n80 = call "LogStatus.vi"("error in (no error)"=w166, "last message"=w183, "message"=w181) -> ("error  out"=w184:errorcluster)  [unwired: 8 in]
        n81 = case shown="Error" w166 {
          tunnel: [_ TRUE] -> w171
          tunnel: [_ "Error"] -> w173
          frame No Error {
          }
          frame Error {
          }
        }
        n82 = Select(t="Initialisation_Record_hardware_serial", s=w163, f="Initialisation_Read_and_check_DDM_EOL_timestamp") -> (s? t:f=w161:string)
      }
      frame "Initialisation_Read_and_check_DDM_EOL_timestamp" {
        n83 = Unbundle By Name(w232) -> ("Table"=w239:string[][], "daemon reference"=w244:refnum<k5>)
        n84 = Unbundle By Name(w217) -> ("MES bool"=w223:refnum<vi>)
        n85 = call "HD_Config.vi"("Step"=enum16{"Initial", "Write", "Read"}."Read") -> ("HD Config out"=w224:T11)  [unwired: 9 in, 1 out]
        n86 = property class="Bool (严格)"(reference=w223) -> ("Value"=w221:bool)  [unwired: 1 in, 2 out]
        n87 = call "Select_Table_Vaule Enable_Disable.vi"("Action"=w240, "Table"=w239) -> ("Enable"=w241:bool)  [unwired: 8 in, 1 out]
        n88 = Unbundle By Name(w224) -> ("Fail_resume_mode"=w222:bool)
        n89 = case shown="False" w241 {
          tunnel: w244 -> [w261 w285]
          tunnel: [TRUE w273] -> w216
          tunnel: [w261 w279] -> w226
          tunnel: [w254 w272] -> w235
          tunnel: w240 -> [w255 w278]
          tunnel: w239 -> [w256 w277]
          tunnel: [_ w275] -> w233
          tunnel: [_ w272] -> _
          tunnel: [w254 w271] -> w213
          tunnel: [w254 w270] -> w231
          tunnel: [w254 w266] -> w230
          tunnel: [w254 w265] -> w229
          tunnel: [w254 w264] -> w228
          tunnel: [w254 w263] -> w227
          frame False {
            w257 = "UIdisplay" ("Process (\"\" - local)")
            w254 = "Skip" ("response")
            n90 = call "Select_Table_Vaule.vi"("Vaule"=w254, "Action"=w255, "Table"=w256) -> ("vaule"=w260:string[])  [unwired: 7 in, 1 out]
            n91 = Build Array (concatenate)(w260, w254, w254) -> (w258:string[])
            n92 = Flatten To XML(anything=w258) -> (xml string=w259:string)
            n93 = call "AMC Send Local Message.vi"("Process (\"\" - local)"=w257, "Message Value"=w259, "Message Name"=w257) -> ()  [unwired: 7 in, 2 out]
          }
          frame True {
            w284 = "UIdisplay" ("Process (\"\" - local)")
            w269 = device_mode."EOL" ("Mode")
            n94 = call "get_cal_info.vi"("Mode"=w269, "daemon reference in"=w285) -> ("error out"=w275:errorcluster, "Parameter"=w268:T13, "response"=w272:string, "daemon reference out"=w279:refnum<k5>)  [unwired: 5 in, 1 out]
            n95 = Number To Decimal String(number=w268) -> (decimal integer string=w267:T14)  [unwired: 1 in]
            n96 = Unbundle By Name(w267) -> ("TIMESTAMP"=w266:string, "RIG_ID"=w265:string, "PASSMARK_ID"=w264:string, "PASSMARK_REV"=w263:string)
            n97 = call "Select_Table_Vaule.vi"("Boolean"=FALSE, "Vaule"=w266, "Action"=w278, "Table"=w277) -> ("Result"=w273:bool, "vaule"=w276:string[])  [unwired: 6 in]
            n98 = case shown="\"EOL\"" w269 {
              tunnel: ["FCT" ("Initialisation.5.3.2.8 Read DDM EOL Timestamp - Mode.Vaule") "EOL" ("Initialisation.5.3.2.8 Read DDM EOL Timestamp - Mode.Vaule") "PROD" ("Initialisation.5.3.2.8 Read DDM EOL Timestamp - Mode.Vaule")] -> w270
              frame "FCT", Default {
              }
              frame "EOL" {
              }
              frame "PROD" {
              }
            }
            n99 = Append True/False String(1:w273, 2:"FAIL" ("真字符串"), 3:"PASS" ("真字符串")) -> (0:w271:string)  [unwired: 1 in]
            n100 = Build Array (concatenate)(w276, w272, w271) -> (w283:string[])
            n101 = Flatten To XML(anything=w283) -> (xml string=w282:string)
            n102 = call "AMC Send Local Message.vi"("Process (\"\" - local)"=w284, "Message Value"=w282, "Message Name"=w284) -> ()  [unwired: 7 in, 2 out]
          }
        }
        n103 = Not(x=w221) -> (.not. x?=w219:bool)
        n104 = Or(x=w222, y=w219) -> (x .or. y?=w220:bool)
        n105 = Select(t=TRUE, s=w220, f=w216) -> (s? t:f=w215:bool)
        n106 = call <vilib>:"Space Constant.vi"() -> ("String"=w243:string)
        n107 = Concatenate Strings(w240, w243, w235) -> (w242:string)
        n108 = case shown="No Error" w233 {
          tunnel: w215 -> [w248 _]
          tunnel: [w249 "Error"] -> w237
          tunnel: [w248 FALSE] -> w236
          frame No Error {
            n109 = Select(t="Initialisation_Read_DDM_SW_version_and_check_before_flashing", s=w248, f="Finalization_NG_unit") -> (s? t:f=w249:string)
          }
          frame Error {
          }
        }
        n110 = Bundle By Name(cluster=w232, "Initialisation.Read DDM EOL Timestamp - Mode"=w231, "Initialisation.Read DDM EOL Timestamp - Timestamp"=w230, "Initialisation.Read DDM EOL Timestamp - Rig ID"=w229, "Initialisation.Read DDM EOL Timestamp - Passmark ID"=w228, "Initialisation.Read DDM EOL Timestamp - Passmark Rev"=w227, "daemon reference"=w226, "Initialisation_Status.Read DDM EOL Timestamp - Mode"=w213, "Initialisation_Status.Read DDM EOL Timestamp - Timestamp"=w213, "Initialisation_Status.Read DDM EOL Timestamp - Rig ID"=w213, "Initialisation_Status.Read DDM EOL Timestamp - Passmark ID"=w213, "Initialisation_Status.Read DDM EOL Timestamp - Passmark Rev"=w213) -> (w234:T1)
        n111 = call "LogStatus.vi"("error in (no error)"=w233, "last message"=w245, "message"=w242) -> ("error  out"=w246:errorcluster)  [unwired: 8 in]
        n112 = Not(x=w236) -> (.not. x?=w238:bool)
      }
      frame "Initialisation_Read_DDM_SW_version_and_check_before_flashing" {
        n113 = Unbundle By Name(w295) -> ("MES bool"=w299:refnum<vi>)
        n114 = Unbundle By Name(w305) -> ("Table"=w310:string[][], "daemon reference"=w316:refnum<k5>)
        n115 = call "HD_Config.vi"("Step"=enum16{"Initial", "Write", "Read"}."Read") -> ("HD Config out"=w300:T11)  [unwired: 9 in, 1 out]
        n116 = property class="Bool (严格)"(reference=w299) -> ("Value"=w297:bool)  [unwired: 1 in, 2 out]
        n117 = Unbundle By Name(w300) -> ("Fail_resume_mode"=w298:bool)
        n118 = Not(x=w297) -> (.not. x?=w296:bool)
        n119 = call "Select_Table_Vaule Enable_Disable.vi"("Action"=w311, "Table"=w310) -> ("Enable"=w312:bool)  [unwired: 8 in, 1 out]
        n120 = case shown="False" w312 {
          tunnel: w316 -> [w327 w339]
          tunnel: [TRUE w334] -> w292
          tunnel: [w327 w338] -> w303
          tunnel: [w326 w330] -> w313
          tunnel: w311 -> [_ w337]
          tunnel: w310 -> [_ w336]
          tunnel: [w326 w330] -> w290
          tunnel: [_ w333] -> w306
          tunnel: [w326 w329] -> w289
          frame False {
            w326 = "Skip" ("software string")
          }
          frame True {
            w344 = "UIdisplay" ("Process (\"\" - local)")
            n121 = call "software_version.vi"("daemon reference in"=w339) -> ("error out"=w333:errorcluster, "software string"=w332:string, "daemon reference out"=w338:refnum<k5>)  [unwired: 7 in, 1 out]
            n122 = Match Pattern(string=w332, regular expression="\\") -> (before substring=w330:string)  [unwired: 1 in, 3 out]
            n123 = call "Select_Table_Vaule.vi"("Vaule"=w330, "Action"=w337, "Table"=w336) -> ("Result"=w334:bool, "vaule"=w335:string[])  [unwired: 7 in]
            n124 = Append True/False String(1:w334, 2:"FAIL" ("真字符串"), 3:"PASS" ("真字符串")) -> (0:w329:string)  [unwired: 1 in]
            n125 = Build Array (concatenate)(w335, w330, w329) -> (w343:string[])
            n126 = Flatten To XML(anything=w343) -> (xml string=w342:string)
            n127 = call "AMC Send Local Message.vi"("Process (\"\" - local)"=w344, "Message Value"=w342, "Message Name"=w344) -> ()  [unwired: 7 in, 2 out]
          }
        }
        n128 = Or(x=w298, y=w296) -> (x .or. y?=w293:bool)
        n129 = call <vilib>:"Space Constant.vi"() -> ("String"=w315:string)
        n130 = Concatenate Strings(w311, w315, w313) -> (w314:string)
        n131 = Select(t=TRUE, s=w293, f=w292) -> (s? t:f=w291:bool)
        n132 = case shown="No Error" w306 {
          tunnel: [w322 "Error"] -> w309
          tunnel: w291 -> [w321 _]
          tunnel: [w321 FALSE ("Result")] -> w307
          frame No Error {
            n133 = Select(t="Initialisation_Read_DDM_serial" ("f"), s=w321, f="Finalization_NG_unit") -> (s? t:f=w322:string)
          }
          frame Error {
          }
        }
        n134 = Bundle By Name(cluster=w305, "Initialisation_Status.Software Version before flashing"=w289, "Initialisation.Software Version before flashing"=w290, "daemon reference"=w303) -> (w304:T1)
        n135 = call "LogStatus.vi"("error in (no error)"=w306, "last message"=w317, "message"=w314) -> ("error  out"=w318:errorcluster)  [unwired: 8 in]
        n136 = Not(x=w307) -> (.not. x?=w308:bool)
      }
      frame "Initialisation_Read_DDM_serial" {
        n137 = Unbundle By Name(w367) -> ("Table"=w347:string[][], "daemon reference"=w377:refnum<k5>, "MES DDM SN"=w354:string)
        n138 = call "Select_Table_Vaule Enable_Disable.vi"("Action"=w372, "Table"=w347) -> ("Enable"=w373:bool)  [unwired: 8 in, 1 out]
        n139 = case shown="True" w373 {
          tunnel: w377 -> [w421 w432]
          tunnel: [w421 w431] -> w365
          tunnel: [w420 w422] -> w374
          tunnel: w372 -> [_ w430]
          tunnel: w347 -> [_ w429]
          tunnel: [w420 w424] -> w351
          tunnel: [_ w427] -> w368
          tunnel: [w420 w426] -> w349
          tunnel: [_ w425] -> w355
          frame False {
            w420 = "Skip" ("software string")
          }
          frame True {
            w437 = "UIdisplay" ("Process (\"\" - local)")
            n140 = call "get_serial.vi"("daemon reference in"=w432) -> ("error out"=w427:errorcluster, "response"=w422:string, "daemon reference out"=w431:refnum<k5>)  [unwired: 7 in, 1 out]
            n141 = call "Select_Table_Vaule.vi"("Vaule"=w422, "Action"=w430, "Table"=w429) -> ("Result"=w425:bool, "vaule"=w428:string[])  [unwired: 7 in]
            n142 = Append True/False String(1:w425, 2:"FAIL" ("真字符串"), 3:"PASS" ("真字符串")) -> (0:w426:string)  [unwired: 1 in]
            n143 = Build Array (concatenate)(w428, w422, w426) -> (w436:string[])
            n144 = Flatten To XML(anything=w436) -> (xml string=w435:string)
            n145 = Concatenate Strings("'" ("字符串"), w422) -> (w424:string)
            n146 = call "AMC Send Local Message.vi"("Process (\"\" - local)"=w437, "Message Value"=w435, "Message Name"=w437) -> ()  [unwired: 7 in, 2 out]
          }
        }
        n147 = Unbundle By Name(w358) -> ("MES bool"=w361:refnum<vi>)
        n148 = call "HD_Config.vi"("Step"=enum16{"Initial", "Write", "Read"}."Read") -> ("HD Config out"=w362:T11)  [unwired: 9 in, 1 out]
        n149 = property class="Bool (严格)"(reference=w361) -> ("Value"=w363:bool)  [unwired: 1 in, 2 out]
        n150 = Unbundle By Name(w362) -> ("Fail_resume_mode"=w360:bool)
        n151 = Not(x=w363) -> (.not. x?=w346:bool)
        n152 = Or(x=w360, y=w346) -> (x .or. y?=w356:bool)
        n153 = call <vilib>:"Space Constant.vi"() -> ("String"=w376:string)
        n154 = String Subset(string=w351, offset (0)=0 ("偏移量(0)"), length (rest)=15 ("长度（剩余）")) -> (substring=w350:string)
        n155 = Concatenate Strings(w372, w376, w374) -> (w375:string)
        n156 = Equal?(x=w350, y=w354) -> (x = y?=w345:bool)
        n157 = Select(t=w355, s=w356, f=w345) -> (s? t:f=w357:bool)
        n158 = case shown="True" w356 {
          tunnel: [w381 w395] -> w348
          tunnel: w357 -> [w389 w392]
          tunnel: w347 -> [w384 w393]
          tunnel: w346 -> [_ w394]
          tunnel: w345 -> [_ w391]
          frame False {
            w388 = "UIdisplay" ("Process (\"\" - local)")
            w382 = "PASS" ("真字符串")
            n159 = call "Select_Table_Vaule.vi"("Vaule"=w382, "Action"="Initialisation_Compare_DDM_serial_MES_SN", "Table"=w384) -> ("vaule"=w385:string[])  [unwired: 7 in, 1 out]
            n160 = Append True/False String(1:w389, 2:"FAIL" ("真字符串"), 3:w382) -> (0:w381:string)  [unwired: 1 in]
            n161 = Build Array (concatenate)(w385, w381, w381) -> (w387:string[])
            n162 = Flatten To XML(anything=w387) -> (xml string=w386:string)
            n163 = call "AMC Send Local Message.vi"("Process (\"\" - local)"=w388, "Message Value"=w386, "Message Name"=w388) -> ()  [unwired: 7 in, 2 out]
          }
          frame True {
            n164 = case shown="True" w394 {
              tunnel: [w397 w406] -> w395
              tunnel: w393 -> [w398 w407]
              tunnel: w392 -> [_ _]
              tunnel: w391 -> [w396 _]
              frame False {
                w404 = "UIdisplay" ("Process (\"\" - local)")
                w399 = "PASS" ("真字符串")
                n165 = call "Select_Table_Vaule.vi"("Vaule"=w399, "Action"="Initialisation_Compare_DDM_serial_MES_SN", "Table"=w398) -> ("vaule"=w401:string[])  [unwired: 7 in, 1 out]
                n166 = Append True/False String(1:w396, 2:"FAIL" ("真字符串"), 3:w399) -> (0:w397:string)  [unwired: 1 in]
                n167 = Build Array (concatenate)(w401, w397, w397) -> (w403:string[])
                n168 = Flatten To XML(anything=w403) -> (xml string=w402:string)
                n169 = call "AMC Send Local Message.vi"("Process (\"\" - local)"=w404, "Message Value"=w402, "Message Name"=w404) -> ()  [unwired: 7 in, 2 out]
              }
              frame True {
                w413 = "UIdisplay" ("Process (\"\" - local)")
                w406 = "Skip" ("output string")
                n170 = call "Select_Table_Vaule.vi"("Vaule"="PASS" ("真字符串"), "Action"="Initialisation_Compare_DDM_serial_MES_SN", "Table"=w407) -> ("vaule"=w410:string[])  [unwired: 7 in, 1 out]
                n171 = Build Array (concatenate)(w410, w406, w406) -> (w412:string[])
                n172 = Flatten To XML(anything=w412) -> (xml string=w411:string)
                n173 = call "AMC Send Local Message.vi"("Process (\"\" - local)"=w413, "Message Value"=w411, "Message Name"=w413) -> ()  [unwired: 7 in, 2 out]
              }
            }
          }
        }
        n174 = case shown="No Error" w368 {
          tunnel: [w415 "Error"] -> w371
          tunnel: w357 -> [w414 _]
          tunnel: [w414 FALSE ("Result")] -> w369
          frame No Error {
            n175 = Select(t="Initialisation_Record_hardware_serial", s=w414, f="Finalization_NG_unit") -> (s? t:f=w415:string)
          }
          frame Error {
          }
        }
        n176 = Bundle By Name(cluster=w367, "Initialisation_Status.Compare DDM SN with MES SN"=w348, "Initialisation_Status.UUT DDM SN"=w349, "Initialisation.Compare DDM SN with MES SN"=w348, "Initialisation.UUT DDM SN"=w350, "daemon reference"=w365) -> (w366:T1)
        n177 = call "LogStatus.vi"("error in (no error)"=w368, "last message"=w378, "message"=w375) -> ("error  out"=w379:errorcluster)  [unwired: 8 in]
        n178 = Not(x=w369) -> (.not. x?=w370:bool)
      }
      frame "Initialisation_Record_hardware_serial" {
        n179 = Unbundle By Name(w450) -> ("Table"=w454:string[][], "daemon reference"=w459:refnum<k5>)
        n180 = call "Select_Table_Vaule Enable_Disable.vi"("Action"=w455, "Table"=w454) -> ("Enable"=w453:bool)  [unwired: 8 in, 1 out]
        n181 = case shown="False" w453 {
          tunnel: w459 -> [w466 w476]
          tunnel: [w466 w475] -> w448
          tunnel: [w465 w470] -> w456
          tunnel: w455 -> [_ w474]
          tunnel: w454 -> [_ w473]
          tunnel: [w465 w469] -> w439
          tunnel: [_ w468] -> w449
          tunnel: [w465 w467] -> w438
          frame False {
            w465 = "Skip" ("software string")
            (unwired) TRUE
          }
          frame True {
            w481 = "UIdisplay" ("Process (\"\" - local)")
            n182 = call "hardware_serial.vi"("daemon reference in"=w476) -> ("error out"=w468:errorcluster, "hardware_serial"=w469:string, "response"=w470:string, "daemon reference out"=w475:refnum<k5>)  [unwired: 6 in, 1 out]
            n183 = call "Select_Table_Vaule.vi"("Vaule"=w470, "Action"=w474, "Table"=w473) -> ("Result"=w471:bool, "vaule"=w472:string[])  [unwired: 7 in]
            n184 = Append True/False String(1:w471, 2:"FAIL" ("真字符串"), 3:"PASS" ("真字符串")) -> (0:w467:string)  [unwired: 1 in]
            n185 = Build Array (concatenate)(w472, w470, w467) -> (w480:string[])
            n186 = Flatten To XML(anything=w480) -> (xml string=w479:string)
            n187 = call "AMC Send Local Message.vi"("Process (\"\" - local)"=w481, "Message Value"=w479, "Message Name"=w481) -> ()  [unwired: 7 in, 2 out]
          }
        }
        n188 = call <vilib>:"Space Constant.vi"() -> ("String"=w458:string)
        n189 = Concatenate Strings(w455, w458, w456) -> (w457:string)
        n190 = Bundle By Name(cluster=w450, "Initialisation_Status.Read Hardware Serial"=w438, "Initialisation.Read Hardware Serial"=w439, "daemon reference"=w448) -> (w447:T1)
        n191 = call "HD_Config.vi"("Step"=enum16{"Initial", "Write", "Read"}."Read") -> ("HD Config out"=w445:T11)  [unwired: 9 in, 1 out]
        n192 = Unbundle By Name(w445) -> ("GRR"=w443:bool)
        n193 = call "LogStatus.vi"("error in (no error)"=w449, "last message"=w460, "message"=w457) -> ("error  out"=w461:errorcluster)  [unwired: 8 in]
        n194 = case shown="Error" w449 {
          tunnel: [_ TRUE] -> w451
          tunnel: [_ "Error"] -> w452
          frame No Error {
          }
          frame Error {
          }
        }
        n195 = Select(t="Initialisation_Read_DDM_SW_Version_and_check_after_flashing", s=w443, f="Initialisation_search_backup_folder_before_flashing_and_check_file_is_exist") -> (s? t:f=w441:string)
      }
      frame "Initialisation_search_backup_folder_before_flashing_and_check_file_is_exist" {
        n196 = Unbundle By Name(w482) -> ("Table"=w491:string[][], "Config"=w484:string[][], "Initialisation.Read Hardware Serial"=w483:string)
        n197 = call "Select_Table_Vaule Enable_Disable.vi"("Action"=w492, "Table"=w491) -> ("Enable"=w490:bool)  [unwired: 8 in, 1 out]
        n198 = case shown="False" w490 {
          tunnel: ["Skip" ("software string") w507] -> w493
          tunnel: w492 -> [_ _]
          tunnel: w491 -> [_ _]
          tunnel: [TRUE ("file or folder exists?") w502] -> w488
          tunnel: w484 -> [_ _]
          tunnel: w483 -> [_ w503]
          frame False {
          }
          frame True {
            n199 = call "PathChoose.vi"(11:PathChoose."backup_before_flashing") -> ("Path_Out"=w505:path)  [unwired: 10 in]
            n200 = List Folder(path=w505) -> (filenames=w504:string[])  [unwired: 3 in, 3 out]
            n201 = for {
              tunnel: w504 -> [w513] mode=indexing
              tunnel: w503 -> [w512]
              tunnel: [w510] -> w502
              stop <- w510 stop-if-true
              n202 = Search and Replace String(input string=w513, search string=w512) -> (number of replacements=w511:i32)  [unwired: 6 in, 3 out]
              n203 = Greater Than 0?(x=w511) -> (x > 0?=w510:bool)
            }
            n204 = Append True/False String(1:w502, 2:"non exist" ("false string"), 3:"exist" ("true string")) -> (0:w507:string)  [unwired: 1 in]
          }
        }
        n205 = call <vilib>:"Space Constant.vi"() -> ("String"=w495:string)
        n206 = Concatenate Strings(w492, w495, w493) -> (w494:string)
        n207 = call "LogStatus.vi"("error in (no error)"=w498, "last message"=w496, "message"=w494) -> ("error  out"=w497:errorcluster)  [unwired: 8 in]
        n208 = Select(t="Initialisation_Flash_SW_follow_SKU", s=w488, f="Initialisation_Backup_DDM_NVM") -> (s? t:f=w485:string)
      }
      frame "Initialisation_Backup_DDM_NVM" {
        n209 = Unbundle By Name(w520) -> ("Table"=w541:string[][], "daemon reference"=w546:refnum<k5>, "Config"=w539:string[][], "Initialisation.Read Hardware Serial"=w522:string)
        n210 = call "PathChoose.vi"(11:PathChoose."backup_before_flashing") -> ("Path_Out"=w529:path)  [unwired: 10 in]
        n211 = Path To String(path=w529) -> (string=w530:string)
        n212 = Format Date/Time String(time format string (%c)="%Y%m%d%H%M%S" ("时间格式字符串(%c)")) -> (date/time string=w531:string)  [unwired: 2 in]
        n213 = call "Select_Table_Vaule Enable_Disable.vi"("Action"=w542, "Table"=w541) -> ("Enable"=w540:bool)  [unwired: 8 in, 1 out]
        n214 = Concatenate Strings(w530, "\\" ("字符串"), w522, "_" ("string"), w531, ".json" ("string")) -> (w528:string)
        n215 = String To Path(string=w528) -> (path=w535:path)
        n216 = call <vilib>:"Check if File or Folder Exists.vi"("path"=w535) -> ("error out"=w533:errorcluster, "file or folder exists?"=w534:bool, "dup path"=w532:path)  [unwired: 8 in]
        n217 = case shown="False" w534 {
          tunnel: w533 -> [w553 w554]
          tunnel: w532 -> [w550 w555]
          tunnel: [w550 w555] -> w521
          tunnel: [w552 w554] -> _
          frame False {
            n218 = Open/Create/Replace File(file path (use dialog)=w550, error in=w553, operation (0:open)=T8."create") -> (error out=w552:errorcluster)  [unwired: 3 in, 2 out]
          }
          frame True {
          }
        }
        n219 = case shown="False" w540 {
          tunnel: w546 -> [w559 w570]
          tunnel: [w559 w569] -> w517
          tunnel: [w558 w560] -> w518
          tunnel: w542 -> [_ w568]
          tunnel: w541 -> [_ w567]
          tunnel: w539 -> [_ _]
          tunnel: [_ w563] -> w536
          tunnel: w521 -> [_ w562]
          tunnel: [w558 w561] -> w514
          tunnel: [w558 w560] -> w515
          frame False {
            w558 = "Skip" ("software string")
            (unwired) TRUE
          }
          frame True {
            w575 = "UIdisplay" ("Process (\"\" - local)")
            n220 = call "backup_nvm.vi"("type"=read_nvm_section."CAL", "File Path"=w562, "daemon reference in"=w570) -> ("error out"=w563:errorcluster, "response"=w560:string, "daemon reference out"=w569:refnum<k5>)  [unwired: 5 in, 1 out]
            n221 = call "Select_Table_Vaule.vi"("Vaule"=w560, "Action"=w568, "Table"=w567) -> ("Result"=w565:bool, "vaule"=w566:string[])  [unwired: 7 in]
            n222 = Append True/False String(1:w565, 2:"FAIL" ("真字符串"), 3:"PASS" ("真字符串")) -> (0:w561:string)  [unwired: 1 in]
            n223 = Build Array (concatenate)(w566, w560, w561) -> (w574:string[])
            n224 = Flatten To XML(anything=w574) -> (xml string=w573:string)
            n225 = call "AMC Send Local Message.vi"("Process (\"\" - local)"=w575, "Message Value"=w573, "Message Name"=w575) -> ()  [unwired: 7 in, 2 out]
          }
        }
        n226 = call <vilib>:"Space Constant.vi"() -> ("String"=w545:string)
        n227 = Concatenate Strings(w542, w545, w518) -> (w544:string)
        n228 = Bundle By Name(cluster=w520, "Initialisation_Status.Backup PCBA Calibration EEPROM Response - CAL"=w514, "Initialisation.Backup PCBA Calibration EEPROM Response - CAL"=w515, "daemon reference"=w517) -> (w519:T1)
        n229 = call "LogStatus.vi"("error in (no error)"=w536, "last message"=w547, "message"=w544) -> ("error  out"=w548:errorcluster)  [unwired: 8 in]
        n230 = case shown="Error" w536 {
          tunnel: [_ TRUE] -> w538
          tunnel: [_ "Error"] -> w537
          frame No Error {
          }
          frame Error {
          }
        }
      }
      frame "Initialisation_Flash_SW_follow_SKU" {
        n231 = Unbundle By Name(w581) -> ("Table"=w594:string[][], "daemon reference"=w598:refnum<k5>, "Config"=w592:string[][])
        n232 = Unbundle By Name(w584) -> ("MainVI"=w583:refnum<vi>)
        n233 = call "Select_Table_Vaule Enable_Disable.vi"("Action"=w595, "Table"=w594) -> ("Enable"=w593:bool)  [unwired: 8 in, 1 out]
        n234 = case shown="True" w593 {
          tunnel: w598 -> [w606 w635]
          tunnel: [w606 w634] -> w579
          tunnel: [w604 w607] -> w582
          tunnel: w595 -> [_ w633]
          tunnel: w594 -> [_ w632]
          tunnel: w592 -> [_ w629]
          tunnel: [TRUE w630] -> w588
          tunnel: string[] ["Initialisation_DDM_Firmware_Hex", "Initialisation_DDM_Firmware_bin", "Initialisation_Flashing_wait_time", "Initialisation_Flashing_Mode", "Initialisation_Product_Mode"] -> [_ w628]
          tunnel: [_ w618] -> w578
          tunnel: w583 -> [_ w616]
          tunnel: [w604 w612] -> w576
          tunnel: [_ w611] -> _
          tunnel: [_ w607] -> _
          tunnel: [_ w609] -> _
          tunnel: [_ w607] -> _
          frame False {
            w604 = "Skip" ("software string")
          }
          frame True {
            w640 = "UIdisplay" ("Process (\"\" - local)")
            n235 = for {
              tunnel: w629 -> [w674]
              tunnel: w628 -> [w673] mode=indexing
              tunnel: [w672] -> w627 mode=indexing
              n236 = call "Index_Config.vi"("Action"=w673, "config"=w674) -> ("data"=w672:string)  [unwired: 9 in]
            }
            n237 = call <vilib>:"Set Busy.vi"("VI reference (current VI)"=w616) -> ("error out"=w617:errorcluster)  [unwired: 9 in, 1 out]
            n238 = Index Array(array=w627) -> (element #1=w626:string, element #2=w608:string, element #3=w611:string, element #4=w613:string, element #5=w614:string)  [unwired: 5 in]
            n239 = String To Path(string=w626) -> (path=w625:path)
            n240 = String To Path(string=w608) -> (path=w624:path)
            n241 = Decimal String To Number(string=w611) -> (number=w623:i32)  [unwired: 2 in, 1 out]
            n242 = Multiply(x=w623, y=1000) -> (x*y=w621:i32)
            n243 = case shown="\"EVT3\", Default" w614 {
              tunnel: w635 -> [w647 w671]
              tunnel: [w648 w670] -> w634
              tunnel: w625 -> [_ w668]
              tunnel: w624 -> [w646 w667]
              tunnel: w621 -> [w644 w666]
              tunnel: [w645 w665] -> w619
              tunnel: [w642 w664] -> w618
              tunnel: w617 -> [w643 w663]
              tunnel: w613 -> [w641 _]
              frame "EVT3", Default {
                n244 = case shown="\"SPC\", Default" w641 {
                  tunnel: [w654 w662] -> w648
                  tunnel: w647 -> [w655 w661]
                  tunnel: w646 -> [w650 w660]
                  tunnel: [w653 w659] -> w645
                  tunnel: w644 -> [w649 w658]
                  tunnel: w643 -> [w651 w657]
                  tunnel: [w652 w656] -> w642
                  frame "SPC", Default {
                    n245 = call "set_product_config_bin.vi"("timeout (25000ms)"=w649, "error in (no error)"=w651, "firmware image bin file"=w650, "daemon reference in"=w655) -> ("error out"=w652:errorcluster, "response"=w653:string, "daemon reference out"=w654:refnum<k5>)  [unwired: 4 in, 1 out]
                  }
                  frame "FF" {
                    n246 = call "flash_firmware_bin.vi"("timeout (25000ms)"=w658, "error in (no error)"=w657, "firmware path"=w660, "daemon reference in"=w661) -> ("error out"=w656:errorcluster, "response"=w659:string, "daemon reference out"=w662:refnum<k5>)  [unwired: 4 in, 1 out]
                  }
                }
              }
              frame "EVT2" {
                n247 = call "flash_firmware.vi"("timeout (25000ms)"=w666, "SW 4.1 and above?"=TRUE, "error in (no error)"=w663, "SIV bin path"=w667, "firmware path"=w668, "daemon reference in"=w671) -> ("error out"=w664:errorcluster, "response"=w665:string, "daemon reference out"=w670:refnum<k5>)  [unwired: 2 in, 1 out]
              }
            }
            n248 = Match Pattern(string=w608, regular expression="data\\") -> (after substring=w609:string)  [unwired: 1 in, 3 out]
            n249 = Match Pattern(string=w619, regular expression="\\") -> (before substring=w607:string)  [unwired: 1 in, 3 out]
            n250 = call "Select_Table_Vaule.vi"("Vaule"=w607, "Action"=w633, "Table"=w632) -> ("Result"=w630:bool, "vaule"=w631:string[])  [unwired: 7 in]
            n251 = call <vilib>:"Unset Busy.vi"("error in (no error)"=w618, "VI reference (current VI)"=w616) -> ("error out"=w615:errorcluster)  [unwired: 9 in]
            n252 = call <vilib>:"Clear Errors.vi"("error in (no error)"=w615) -> ()  [unwired: 5 in, 2 out]
            n253 = Append True/False String(1:w630, 2:"FAIL" ("真字符串"), 3:"PASS" ("真字符串")) -> (0:w612:string)  [unwired: 1 in]
            n254 = Build Array (concatenate)(w631, w607, w612) -> (w639:string[])
            n255 = Flatten To XML(anything=w639) -> (xml string=w638:string)
            n256 = call "AMC Send Local Message.vi"("Process (\"\" - local)"=w640, "Message Value"=w638, "Message Name"=w640) -> ()  [unwired: 7 in, 2 out]
          }
        }
        n257 = call <vilib>:"Space Constant.vi"() -> ("String"=w597:string)
        n258 = Concatenate Strings(w595, w597, w582) -> (w596:string)
        n259 = Bundle By Name(cluster=w581, "daemon reference"=w579, "Initialisation.Flash Firmware Version"=w576, "Initialisation_Status.Flash Firmware Version"=w576) -> (w580:T1)
        n260 = call "LogStatus.vi"("error in (no error)"=w578, "last message"=w599, "message"=w596) -> ("error  out"=w600:errorcluster)  [unwired: 8 in]
        n261 = Select(t="Initialisation_Read_DDM_SW_Version_and_check_after_flashing", s=w588, f="Reflashing") -> (s? t:f=w589:string)
        n262 = case shown="Error" w578 {
          tunnel: [_ TRUE] -> w585
          tunnel: [_ "Error"] -> w586
          frame No Error {
          }
          frame Error {
          }
        }
      }
      frame "Initialisation_Read_DDM_SW_Version_and_check_after_flashing" {
        n263 = Unbundle By Name(w682) -> ("MES bool"=w685:refnum<vi>)
        n264 = Unbundle By Name(w694) -> ("Table"=w699:string[][], "daemon reference"=w704:refnum<k5>, "Config"=w697:string[][])
        n265 = call "HD_Config.vi"("Step"=enum16{"Initial", "Write", "Read"}."Read") -> ("HD Config out"=w684:T11)  [unwired: 9 in, 1 out]
        n266 = property class="Bool (严格)"(reference=w685) -> ("Value"=w687:bool)  [unwired: 1 in, 2 out]
        n267 = Unbundle By Name(w684) -> ("GRR"=w678:bool, "Fail_resume_mode"=w686:bool)
        n268 = call "Select_Table_Vaule Enable_Disable.vi"("Action"=w700, "Table"=w699) -> ("Enable"=w698:bool)  [unwired: 8 in, 1 out]
        n269 = Not(x=w687) -> (.not. x?=w688:bool)
        n270 = case shown="True" w698 {
          tunnel: w704 -> [w719 w727]
          tunnel: [w719 w726] -> w691
          tunnel: [w717 w721] -> w701
          tunnel: w700 -> [_ w730]
          tunnel: w699 -> [_ w729]
          tunnel: w697 -> [_ _]
          tunnel: [TRUE w725] -> w680
          tunnel: [w717 w721] -> w675
          tunnel: [_ w724] -> w693
          tunnel: [w717 w720] -> w676
          frame False {
            w717 = "Skip" ("software string")
          }
          frame True {
            w735 = "UIdisplay" ("Process (\"\" - local)")
            n271 = call "software_version.vi"("daemon reference in"=w727) -> ("error out"=w724:errorcluster, "software string"=w722:string, "daemon reference out"=w726:refnum<k5>)  [unwired: 7 in, 1 out]
            n272 = Match Pattern(string=w722, regular expression="\\") -> (before substring=w721:string)  [unwired: 1 in, 3 out]
            n273 = call "Select_Table_Vaule.vi"("Vaule"=w721, "Action"=w730, "Table"=w729) -> ("Result"=w725:bool, "vaule"=w728:string[])  [unwired: 7 in]
            n274 = Append True/False String(1:w725, 2:"FAIL" ("真字符串"), 3:"PASS" ("真字符串")) -> (0:w720:string)  [unwired: 1 in]
            n275 = Build Array (concatenate)(w728, w721, w720) -> (w734:string[])
            n276 = Flatten To XML(anything=w734) -> (xml string=w733:string)
            n277 = call "AMC Send Local Message.vi"("Process (\"\" - local)"=w735, "Message Value"=w733, "Message Name"=w735) -> ()  [unwired: 7 in, 2 out]
          }
        }
        n278 = Or(x=w686, y=w688) -> (x .or. y?=w690:bool)
        n279 = call <vilib>:"Space Constant.vi"() -> ("String"=w703:string)
        n280 = Select(t=TRUE, s=w690, f=w680) -> (s? t:f=w681:bool)
        n281 = Concatenate Strings(w700, w703, w701) -> (w702:string)
        n282 = case shown="No Error" w693 {
          tunnel: [w712 "Error"] -> w696
          tunnel: w681 -> [w708 _]
          tunnel: [w710 FALSE ("Result")] -> w677
          tunnel: w678 -> [w709 _]
          frame No Error {
            w711 = "Initialisation_Set_SKU_Config_base_on_variant"
            n283 = Select(t=w709, s=w709, f=w708) -> (s? t:f=w710:bool)
            n284 = Select(t=w711, s=w708, f="Finalization_NG_unit") -> (s? t:f=w713:string)
            n285 = Select(t=w711, s=w709, f=w713) -> (s? t:f=w712:string)
          }
          frame Error {
          }
        }
        n286 = Bundle By Name(cluster=w694, "daemon reference"=w691, "Initialisation.Check SW Version"=w675, "Initialisation.Read DDM SW Version after flashing"=w675, "Initialisation_Status.Check SW Version"=w676, "Initialisation_Status.Read DDM SW Version after flashing"=w676) -> (w692:T1)
        n287 = call "LogStatus.vi"("error in (no error)"=w693, "last message"=w705, "message"=w702) -> ("error  out"=w706:errorcluster)  [unwired: 8 in]
        n288 = Not(x=w677) -> (.not. x?=w695:bool)
      }
      frame "Initialisation_Set_SKU_Config_base_on_variant" {
        # "文件与LMT调用文件一样.mem文件"
        n289 = Unbundle By Name(w748) -> ("Table"=w755:string[][], "daemon reference"=w759:refnum<k5>, "Config"=w753:string[][])
        n290 = call "Select_Table_Vaule Enable_Disable.vi"("Action"=w756, "Table"=w755) -> ("Enable"=w754:bool)  [unwired: 8 in, 1 out]
        n291 = case shown="True" w754 {
          tunnel: w759 -> [w767 w782]
          tunnel: [w767 w781] -> w746
          tunnel: [w765 w771] -> w750
          tunnel: w756 -> [_ w786]
          tunnel: w755 -> [_ w785]
          tunnel: w753 -> [_ w780]
          tunnel: [TRUE w783] -> _
          tunnel: string[] ["Initialisation_SKU_Config_Hex", "Initialisation_SKU_ID"] -> [_ w778]
          tunnel: [_ w779] -> w747
          tunnel: [w765 w775] -> w736
          tunnel: [w765 w774] -> w737
          tunnel: [_ w772] -> _
          frame False {
            w765 = "Skip" ("software string")
          }
          frame True {
            w791 = "UIdisplay" ("Process (\"\" - local)")
            n292 = for {
              tunnel: w780 -> [w794]
              tunnel: w778 -> [w793] mode=indexing
              tunnel: [w792] -> w777 mode=indexing
              n293 = call "Index_Config.vi"("Action"=w793, "config"=w794) -> ("data"=w792:string)  [unwired: 9 in]
            }
            n294 = Index Array(array=w777) -> (element #1=w770:string, element #2=w772:string)  [unwired: 2 in]
            n295 = String To Path(string=w770) -> (path=w776:path)
            n296 = Match Pattern(string=w770, regular expression="data\\" ("正则表达式")) -> (after substring=w768:string)  [unwired: 1 in, 3 out]
            n297 = call "set_sku.vi"("SKU ID"=w772, "sku hex filepath"=w776, "daemon reference in"=w782) -> ("error out"=w779:errorcluster, "response"=w774:string, "daemon reference out"=w781:refnum<k5>)  [unwired: 5 in, 1 out]
            n298 = call <vilib>:"Space Constant.vi"() -> ("String"=w769:string)
            n299 = call "Select_Table_Vaule.vi"("Vaule"=w774, "Action"=w786, "Table"=w785) -> ("Result"=w783:bool, "vaule"=w784:string[])  [unwired: 7 in]
            n300 = Concatenate Strings(w768, w769, w774) -> (w771:string)
            n301 = Append True/False String(1:w783, 2:"FAIL" ("真字符串"), 3:"PASS" ("真字符串")) -> (0:w775:string)  [unwired: 1 in]
            n302 = Build Array (concatenate)(w784, w771, w775) -> (w790:string[])
            n303 = Flatten To XML(anything=w790) -> (xml string=w789:string)
            n304 = call "AMC Send Local Message.vi"("Process (\"\" - local)"=w791, "Message Value"=w789, "Message Name"=w791) -> ()  [unwired: 7 in, 2 out]
          }
        }
        n305 = call <vilib>:"Space Constant.vi"() -> ("String"=w758:string)
        n306 = Concatenate Strings(w756, w758, w750) -> (w757:string)
        n307 = Bundle By Name(cluster=w748, "Initialisation_Status.Set SKU Config"=w736, "Initialisation.Set SKU Config"=w737, "daemon reference"=w746) -> (w745:T1)
        n308 = call "HD_Config.vi"("Step"=enum16{"Initial", "Write", "Read"}."Read") -> ("HD Config out"=w741:T11)  [unwired: 9 in, 1 out]
        n309 = Unbundle By Name(w741) -> ("GRR"=w743:bool)
        n310 = call "LogStatus.vi"("error in (no error)"=w747, "last message"=w760, "message"=w757) -> ("error  out"=w761:errorcluster)  [unwired: 8 in]
        n311 = case shown="Error" w747 {
          tunnel: [_ TRUE] -> w751
          tunnel: [_ "Error"] -> w752
          frame No Error {
          }
          frame Error {
          }
        }
        n312 = Select(t="Initialisation_Set_DDM_to_EOL_Mode", s=w743, f="Initialisation_Get_and_check_UUT_Ready_Status") -> (s? t:f=w739:string)
      }
      frame "Initialisation_Get_and_check_UUT_Ready_Status" {
        n313 = Unbundle By Name(w812) -> ("Table"=w819:string[][], "daemon reference"=w823:refnum<k5>, "Config"=w817:string[][])
        n314 = Unbundle By Name(w802) -> ("MES bool"=w805:refnum<vi>)
        n315 = call "HD_Config.vi"("Step"=enum16{"Initial", "Write", "Read"}."Read") -> ("HD Config out"=w804:T11)  [unwired: 9 in, 1 out]
        n316 = property class="Bool (严格)"(reference=w805) -> ("Value"=w807:bool)  [unwired: 1 in, 2 out]
        n317 = Unbundle By Name(w804) -> ("Fail_resume_mode"=w806:bool)
        n318 = call "Select_Table_Vaule Enable_Disable.vi"("Action"=w820, "Table"=w819) -> ("Enable"=w818:bool)  [unwired: 8 in, 1 out]
        n319 = case shown="False" w818 {
          tunnel: w823 -> [w842 w847]
          tunnel: [w842 w846] -> w798
          tunnel: ["Skip" ("software string") w844] -> w813
          tunnel: w820 -> [w834 w851]
          tunnel: w819 -> [w835 w850]
          tunnel: w817 -> [_ _]
          tunnel: [TRUE w848] -> w800
          tunnel: [_ w845] -> w799
          tunnel: [w833 w844] -> w796
          tunnel: [w833 w843] -> w795
          frame False {
            w839 = "UIdisplay" ("Process (\"\" - local)")
            w833 = "Skip" ("Action")
            n320 = call "Select_Table_Vaule.vi"("Vaule"=w833, "Action"=w834, "Table"=w835) -> ("vaule"=w836:string[])  [unwired: 7 in, 1 out]
            n321 = Build Array (concatenate)(w836, w833, w833) -> (w838:string[])
            n322 = Flatten To XML(anything=w838) -> (xml string=w837:string)
            n323 = call "AMC Send Local Message.vi"("Process (\"\" - local)"=w839, "Message Value"=w837, "Message Name"=w839) -> ()  [unwired: 7 in, 2 out]
          }
          frame True {
            w856 = "UIdisplay" ("Process (\"\" - local)")
            n324 = call "ready_status.vi"("daemon reference in"=w847) -> ("error out"=w845:errorcluster, "response"=w844:string, "daemon reference out"=w846:refnum<k5>)  [unwired: 7 in, 1 out]
            n325 = call "Select_Table_Vaule.vi"("Vaule"=w844, "Action"=w851, "Table"=w850) -> ("Result"=w848:bool, "vaule"=w849:string[])  [unwired: 7 in]
            n326 = Append True/False String(1:w848, 2:"FAIL" ("真字符串"), 3:"PASS" ("真字符串")) -> (0:w843:string)  [unwired: 1 in]
            n327 = Build Array (concatenate)(w849, w844, w843) -> (w855:string[])
            n328 = Flatten To XML(anything=w855) -> (xml string=w854:string)
            n329 = call "AMC Send Local Message.vi"("Process (\"\" - local)"=w856, "Message Value"=w854, "Message Name"=w856) -> ()  [unwired: 7 in, 2 out]
          }
        }
        n330 = Not(x=w807) -> (.not. x?=w808:bool)
        n331 = Or(x=w806, y=w808) -> (x .or. y?=w810:bool)
        n332 = Select(t=TRUE, s=w810, f=w800) -> (s? t:f=w801:bool)
        n333 = call <vilib>:"Space Constant.vi"() -> ("String"=w822:string)
        n334 = Concatenate Strings(w820, w822, w813) -> (w821:string)
        n335 = case shown="No Error" w799 {
          tunnel: [w828 "Error"] -> w816
          tunnel: w801 -> [w827 _]
          tunnel: [w827 FALSE ("Result")] -> w814
          frame No Error {
            n336 = Select(t="Initialisation_Set_DDM_to_EOL_Mode", s=w827, f="Finalization_NG_unit") -> (s? t:f=w828:string)
          }
          frame Error {
          }
        }
        n337 = Bundle By Name(cluster=w812, "Initialisation_Status.Ready Status"=w795, "Initialisation.Ready Status"=w796, "daemon reference"=w798) -> (w811:T1)
        n338 = call "LogStatus.vi"("error in (no error)"=w799, "last message"=w824, "message"=w821) -> ("error  out"=w825:errorcluster)  [unwired: 8 in]
        n339 = Not(x=w814) -> (.not. x?=w815:bool)
      }
      frame "Initialisation_Set_DDM_to_EOL_Mode" {
        n340 = Unbundle By Name(w864) -> ("Table"=w872:string[][], "daemon reference"=w876:refnum<k5>, "Config"=w870:string[][])
        n341 = call "Select_Table_Vaule Enable_Disable.vi"("Action"=w873, "Table"=w872) -> ("Enable"=w871:bool)  [unwired: 8 in, 1 out]
        n342 = case shown="False" w871 {
          tunnel: w876 -> [w888 w895]
          tunnel: [w888 w894] -> w866
          tunnel: [w886 w892] -> w869
          tunnel: w873 -> [_ w899]
          tunnel: w872 -> [_ w898]
          tunnel: w870 -> [_ _]
          tunnel: [TRUE w896] -> _
          tunnel: [_ w893] -> w868
          tunnel: [_ w892] -> _
          tunnel: [w886 w891] -> w857
          tunnel: [w886 w889] -> w858
          frame False {
            w886 = "Skip" ("software string")
          }
          frame True {
            w890 = device_mode."EOL" ("Mode")
            w904 = "UIdisplay" ("Process (\"\" - local)")
            n343 = call "set_device_mode.vi"("Mode"=w890, "daemon reference in"=w895) -> ("error out"=w893:errorcluster, "response"=w892:string, "daemon reference out"=w894:refnum<k5>)  [unwired: 6 in, 1 out]
            n344 = call "Select_Table_Vaule.vi"("Vaule"=w892, "Action"=w899, "Table"=w898) -> ("Result"=w896:bool, "vaule"=w897:string[])  [unwired: 7 in]
            n345 = case shown="\"EOL\"" w890 {
              tunnel: ["FCT" ("Initialisation.5.3.2.8 Read DDM EOL Timestamp - Mode.Vaule") "EOL" ("Initialisation.5.3.2.8 Read DDM EOL Timestamp - Mode.Vaule") "PROD" ("Initialisation.5.3.2.8 Read DDM EOL Timestamp - Mode.Vaule")] -> w889
              frame "FCT", Default {
              }
              frame "EOL" {
              }
              frame "PROD" {
              }
            }
            n346 = call "Time Delay"("error in (no error)"=w893) -> ()  [unwired: 10 in, 1 out]
            n347 = Append True/False String(1:w896, 2:"FAIL" ("真字符串"), 3:"PASS" ("真字符串")) -> (0:w891:string)  [unwired: 1 in]
            n348 = Build Array (concatenate)(w897, w892, w891) -> (w903:string[])
            n349 = Flatten To XML(anything=w903) -> (xml string=w902:string)
            n350 = call "AMC Send Local Message.vi"("Process (\"\" - local)"=w904, "Message Value"=w902, "Message Name"=w904) -> ()  [unwired: 7 in, 2 out]
          }
        }
        n351 = call <vilib>:"Space Constant.vi"() -> ("String"=w875:string)
        n352 = Concatenate Strings(w873, w875, w869) -> (w874:string)
        n353 = call "HD_Config.vi"("Step"=enum16{"Initial", "Write", "Read"}."Read") -> ("HD Config out"=w862:T11)  [unwired: 9 in, 1 out]
        n354 = Unbundle By Name(w862) -> ("GRR"=w859:bool)
        n355 = case shown="No Error" w868 {
          tunnel: [w880 TRUE] -> w863
          tunnel: [w883 "Error"] -> w860
          tunnel: w859 -> [w880 _]
          frame No Error {
            n356 = Select(t="Power_Tunings_and_AW_Performance_Test", s=w880, f="Initialisation_Get_and_check_DDM_Parameter") -> (s? t:f=w883:string)
          }
          frame Error {
          }
        }
        n357 = Bundle By Name(cluster=w864, "Initialisation_Status.Set Device Mode to EOL"=w857, "Initialisation.Set Device Mode to EOL"=w858, "daemon reference"=w866) -> (w867:T1)
        n358 = call "LogStatus.vi"("error in (no error)"=w868, "last message"=w877, "message"=w874) -> ("error  out"=w878:errorcluster)  [unwired: 8 in]
      }
      frame "Initialisation_Get_and_check_DDM_Parameter" {
        n359 = Unbundle By Name(w927) -> ("Table"=w934:string[][], "daemon reference"=w939:refnum<k5>, "Config"=w932:string[][])
        n360 = call "Select_Table_Vaule Enable_Disable.vi"("Action"=w935, "Table"=w934) -> ("Enable"=w933:bool)  [unwired: 8 in, 1 out]
        n361 = case shown="True" w933 {
          tunnel: w939 -> [w948 w977]
          tunnel: [w948 w976] -> w913
          tunnel: [w947 w968] -> w936
          tunnel: w935 -> [_ w974]
          tunnel: w934 -> [_ w978]
          tunnel: w932 -> [_ _]
          tunnel: [_ w967] -> w925
          tunnel: T10[] ["voltage", "current", "power", "speed", "pressure"] ("Parameter") -> [_ w963]
          tunnel: [w946 w955] -> w926
          tunnel: [w946 w954] -> w923
          tunnel: [_ w953] -> w920
          tunnel: [_ w949] -> w919
          frame False {
            w947 = "Skip" ("software string")
            n362 = Initialize Array(w947, 5 ("维数大小")) -> (w946:string[])
          }
          frame True {
            w972 = string[] ["Initialisation_DDM_Voltage", "Initialisation_DDM_Current", "Initialisation_DDM_Power", "Initialisation_DDM_Speed", "Initialisation_DDM_Pressure"]
            n363 = for {
              tunnel: [w984] -> w962 mode=indexing
              tunnel: [w983] -> w967
              tunnel: [w979] -> w964 mode=indexing
              shift-right: [w985] -> w976
              shift-left: w977 -> [w986]
              tunnel: w963 -> [w980] mode=indexing
              n364 = Build Array(w980) -> (w981:T10[])
              n365 = call "get_parameter.vi"("Parameter"=w981, "daemon reference in"=w986) -> ("error out"=w983:errorcluster, "response"=w984:string, "values"=w982:dbl[], "daemon reference out"=w985:refnum<k5>)  [unwired: 5 in, 1 out]
              n366 = Index Array(array=w982) -> (element=w979:dbl)  [unwired: 1 in]
            }
            n367 = in-place {
              w991 = 1000.0
              n368 = in-place-array #1(w964, 3, 4) -> (w990:dbl, w987:dbl)
              n369 = Divide(x=w990, y=w991) -> (x/y=w989:dbl)
              n370 = Divide(x=w987, y=w991) -> (x/y=w988:dbl)
              n371 = in-place-array #1(w989, w988) -> (w953:dbl[])  [unwired: 2 out]
            }
            n372 = Array To Spreadsheet String(delimiter (Tab)=",", array=w962, 3:"" ("format string")) -> (spreadsheet string=w961:string)
            n373 = Build Array (concatenate)(w974, w972) -> (w975:string[])
            n374 = Number To Fractional String(number=w953) -> (F-format string=w954:string[])  [unwired: 3 in]
            n375 = Interleave 1D Arrays(w972, w954) -> (w971:string[])
            n376 = Build Array (concatenate)(w961, w954) -> (w973:string[])
            n377 = Array To Spreadsheet String(delimiter (Tab)=";" ("分隔符(Tab)"), array=w971, 3:"" ("格式字符串")) -> (spreadsheet string=w968:string)
            n378 = for {
              tunnel: w978 -> [w998]
              tunnel: w973 -> [w996] mode=indexing
              tunnel: w975 -> [w995] mode=indexing
              tunnel: [w993] -> w956 mode=indexing
              tunnel: [w992] -> w950 mode=indexing
              w1003 = "UIdisplay" ("Process (\"\" - local)")
              n379 = call "Select_Table_Vaule.vi"("Boolean"=TRUE, "Vaule"=w996, "Action"=w995, "Table"=w998) -> ("Result"=w992:bool, "vaule"=w997:string[])  [unwired: 6 in]
              n380 = Append True/False String(1:w992, 2:"FAIL" ("真字符串"), 3:"PASS" ("真字符串")) -> (0:w993:string)  [unwired: 1 in]
              n381 = Build Array (concatenate)(w997, w996, w993) -> (w1002:string[])
              n382 = Flatten To XML(anything=w1002) -> (xml string=w1001:string)
              n383 = call "AMC Send Local Message.vi"("Process (\"\" - local)"=w1003, "Message Value"=w1001, "Message Name"=w1003) -> ()  [unwired: 7 in, 2 out]
            }
            n384 = Delete From Array(array=w950, length=1 ("长度"), index=0 ("索引")) -> (array with subset deleted=w949:bool[])  [unwired: 1 out]
            n385 = Delete From Array(array=w956, length=1 ("长度"), index=0 ("索引")) -> (array with subset deleted=w955:string[])  [unwired: 1 out]
          }
        }
        n386 = call <vilib>:"Space Constant.vi"() -> ("String"=w938:string)
        n387 = Concatenate Strings(w935, w938, w936) -> (w937:string)
        n388 = Index Array(array=w923) -> (element #1=w914:string, element #2=w915:string, element #3=w916:string, element #4=w917:string, element #5=w918:string)  [unwired: 5 in]
        n389 = Index Array(array=w926) -> (element #1=w912:string, element #2=w911:string, element #3=w910:string, element #4=w909:string, element #5=w908:string)  [unwired: 5 in]
        n390 = Bundle By Name(cluster=w927, "daemon reference"=w913, "Initialisation.DDM Parameter - Voltage"=w914, "Initialisation.DDM Parameter - Current"=w915, "Initialisation.DDM Parameter - Power"=w916, "Initialisation.DDM Parameter - Speed"=w917, "Initialisation.DDM Parameter - Pressure"=w918, "Initialisation_Status.DDM Parameter - Voltage"=w912, "Initialisation_Status.DDM Parameter - Current"=w911, "Initialisation_Status.DDM Parameter - Power"=w910, "Initialisation_Status.DDM Parameter - Speed"=w909, "Initialisation_Status.DDM Parameter - Pressure"=w908) -> (w924:T1)
        n391 = Bundle By Name(cluster=w922, "Initialisation.DDM_Parameter"=w920, "Initialisation.DDM_Parameter_status"=w919) -> (w921:T3)
        n392 = call "LogStatus.vi"("error in (no error)"=w925, "last message"=w940, "message"=w937) -> ("error  out"=w941:errorcluster)  [unwired: 8 in]
        n393 = case shown="Error" w925 {
          tunnel: [_ TRUE] -> w929
          tunnel: [_ "Error"] -> w930
          frame No Error {
          }
          frame Error {
          }
        }
      }
      frame "Initialisation_Get_and_check_Tester_Parameter" {
        n394 = Unbundle By Name(w1022) -> ("Table"=w1026:string[][], "daemon reference"=w1031:refnum<k5>, "Config"=w1024:string[][])
        n395 = call "Select_Table_Vaule Enable_Disable.vi"("Action"=w1027, "Table"=w1026) -> ("Enable"=w1025:bool)  [unwired: 8 in, 1 out]
        n396 = case shown="False" w1025 {
          tunnel: w1031 -> [w1039 w1061]
          tunnel: [w1039 w1061] -> w1020
          tunnel: [w1038 w1052] -> w1028
          tunnel: w1027 -> [_ w1059]
          tunnel: w1026 -> [_ w1062]
          tunnel: w1024 -> [_ _]
          tunnel: [w1037 w1051] -> w1018
          tunnel: [w1037 w1046] -> w1021
          tunnel: [_ w1045] -> _
          tunnel: [_ w1044] -> w1015
          tunnel: [_ w1040] -> w1014
          frame False {
            w1038 = "Skip" ("software string")
            n397 = Initialize Array(w1038, 5 ("维数大小")) -> (w1037:string[])
          }
          frame True {
            w1056 = string[] ["Initialisation_PM_Voltage", "Initialisation_PM_Current", "Initialisation_PM_Power", "Initialisation_Ambient_Pressure", "Initialisation_Ambient_Temperature", "Initialisation_Tester_Reference_Ambient_Pressure"]
            n398 = call "Initialisation_Tester_Parameter.vi"() -> ("Pressure(Pa)"=w1050:dbl, "Initialisation_Tester_Parameter"=w1044:dbl[])  [unwired: 10 in]
            n399 = Number To Fractional String(number=w1044) -> (F-format string=w1051:string[])  [unwired: 3 in]
            n400 = Number To Fractional String(number=w1050) -> (F-format string=w1045:string)  [unwired: 3 in]
            n401 = Interleave 1D Arrays(w1056, w1051) -> (w1055:string[])
            n402 = Array To Spreadsheet String(delimiter (Tab)=";" ("分隔符(Tab)"), array=w1055, 3:"" ("格式字符串")) -> (spreadsheet string=w1052:string)
            n403 = Build Array (concatenate)(w1059, w1056) -> (w1060:string[])
            n404 = Build Array (concatenate)("", w1051) -> (w1058:string[])
            n405 = for {
              tunnel: w1062 -> [w1069]
              tunnel: w1058 -> [w1067] mode=indexing
              tunnel: w1060 -> [w1066] mode=indexing
              tunnel: [w1064] -> w1049 mode=indexing
              tunnel: [w1063] -> w1041 mode=indexing
              w1074 = "UIdisplay" ("Process (\"\" - local)")
              n406 = call "Select_Table_Vaule.vi"("Boolean"=TRUE, "Vaule"=w1067, "Action"=w1066, "Table"=w1069) -> ("Result"=w1063:bool, "vaule"=w1068:string[])  [unwired: 6 in]
              n407 = Append True/False String(1:w1063, 2:"FAIL" ("真字符串"), 3:"PASS" ("真字符串")) -> (0:w1064:string)  [unwired: 1 in]
              n408 = Build Array (concatenate)(w1068, w1067, w1064) -> (w1073:string[])
              n409 = Flatten To XML(anything=w1073) -> (xml string=w1072:string)
              n410 = call "AMC Send Local Message.vi"("Process (\"\" - local)"=w1074, "Message Value"=w1072, "Message Name"=w1074) -> ()  [unwired: 7 in, 2 out]
            }
            n411 = Delete From Array(array=w1041, length=1 ("长度"), index=0 ("索引")) -> (array with subset deleted=w1040:bool[])  [unwired: 1 out]
            n412 = Delete From Array(array=w1049, length=1 ("长度"), index=0 ("索引")) -> (array with subset deleted=w1046:string[])  [unwired: 1 out]
          }
        }
        n413 = call <vilib>:"Space Constant.vi"() -> ("String"=w1030:string)
        n414 = Concatenate Strings(w1027, w1030, w1028) -> (w1029:string)
        n415 = Index Array(array=w1021) -> (element #1=w1008:string, element #2=w1007:string, element #3=w1006:string, element #4=w1005:string, element #5=w1004:string)  [unwired: 5 in]
        n416 = Index Array(array=w1018) -> (element #1=w1013:string, element #2=w1012:string, element #3=w1011:string, element #4=w1010:string, element #5=w1009:string)  [unwired: 5 in]
        n417 = Bundle By Name(cluster=w1022, "daemon reference"=w1020, "Initialisation.Tester Parameter - Voltage"=w1013, "Initialisation.Tester Parameter - Current"=w1012, "Initialisation.Tester Parameter - Power"=w1011, "Initialisation.Tester Parameter - Ambient Pressure"=w1010, "Initialisation.Tester Parameter - Ambient Temperature"=w1009, "Initialisation_Status.Tester Parameter - Voltage"=w1008, "Initialisation_Status.Tester Parameter - Current"=w1007, "Initialisation_Status.Tester Parameter - Power"=w1006, "Initialisation_Status.Tester Parameter - Ambient Pressure"=w1005, "Initialisation_Status.Tester Parameter - Ambient Temperature"=w1004) -> (w1019:T1)
        n418 = Bundle By Name(cluster=w1017, "Initialisation.Get_Tester_Parameter"=w1015, "Initialisation.Get_Tester_Parameter_status"=w1014) -> (w1016:T3)
        n419 = call "LogStatus.vi"("error in (no error)"=w1034, "last message"=w1032, "message"=w1029) -> ("error  out"=w1033:errorcluster)  [unwired: 8 in]
      }
      frame "Initialisation_Calculate_and_check_tester_parameter" {
        n420 = Unbundle By Name(w1100) -> ("Initialisation.DDM_Parameter"=w1099:dbl[], "Initialisation.Get_Tester_Parameter"=w1098:dbl[])
        n421 = Unbundle By Name(w1096) -> ("Table"=w1111:string[][], "daemon reference"=w1117:refnum<k5>, "Config"=w1109:string[][])
        n422 = call "Select_Table_Vaule Enable_Disable.vi"("Action"=w1112, "Table"=w1111) -> ("Enable"=w1110:bool)  [unwired: 8 in, 1 out]
        n423 = case shown="False" w1110 {
          tunnel: w1117 -> [w1125 w1147]
          tunnel: [w1125 w1147] -> w1095
          tunnel: [w1124 w1138] -> w1113
          tunnel: w1112 -> [_ w1145]
          tunnel: w1111 -> [_ w1148]
          tunnel: w1109 -> [_ _]
          tunnel: [_ w1137] -> w1101
          tunnel: w1099 -> [_ w1136]
          tunnel: w1098 -> [_ w1135]
          tunnel: [_ w1131] -> w1097
          tunnel: [w1123 w1127] -> w1075
          tunnel: [w1123 w1126] -> w1076
          frame False {
            w1124 = "Skip" ("software string")
            n424 = Initialize Array(w1124, 3 ("维数大小")) -> (w1123:string[])
          }
          frame True {
            w1139 = string[] ["Initialisation_DDM_Pressure_corrected", "Initialisation_DDM_Real_Power", "Initialisation_Delta_V"]
            n425 = call "AW_Calculate_Tester_Parameter_Initialisation.vi"("Tester Parameter"=w1135, "DDM Parameter"=w1136) -> ("Calculate Tester Parameter"=w1137:dbl[])  [unwired: 9 in]
            n426 = Number To Fractional String(number=w1137) -> (F-format string=w1126:string[])  [unwired: 3 in]
            n427 = Interleave 1D Arrays(w1139, w1126) -> (w1142:string[])
            n428 = Array To Spreadsheet String(delimiter (Tab)=";" ("分隔符(Tab)"), array=w1142, 3:"" ("格式字符串")) -> (spreadsheet string=w1138:string)
            n429 = Build Array (concatenate)(w1145, w1139) -> (w1146:string[])
            n430 = Build Array (concatenate)("", w1126) -> (w1144:string[])
            n431 = for {
              tunnel: w1148 -> [w1154]
              tunnel: w1144 -> [w1152] mode=indexing
              tunnel: w1146 -> [w1151] mode=indexing
              tunnel: [w1150] -> w1134 mode=indexing
              tunnel: [w1149] -> w1128 mode=indexing
              w1159 = "UIdisplay" ("Process (\"\" - local)")
              n432 = call "Select_Table_Vaule.vi"("Vaule"=w1152, "Action"=w1151, "Table"=w1154) -> ("Result"=w1150:bool, "vaule"=w1153:string[])  [unwired: 7 in]
              n433 = Append True/False String(1:w1150, 2:"FAIL" ("真字符串"), 3:"PASS" ("真字符串")) -> (0:w1149:string)  [unwired: 1 in]
              n434 = Build Array (concatenate)(w1153, w1152, w1149) -> (w1158:string[])
              n435 = Flatten To XML(anything=w1158) -> (xml string=w1157:string)
              n436 = call "AMC Send Local Message.vi"("Process (\"\" - local)"=w1159, "Message Value"=w1157, "Message Name"=w1159) -> ()  [unwired: 7 in, 2 out]
            }
            n437 = Delete From Array(array=w1134, length=1 ("长度"), index=0 ("索引")) -> (array with subset deleted=w1131:bool[])  [unwired: 1 out]
            n438 = Delete From Array(array=w1128, length=1 ("长度"), index=0 ("索引")) -> (array with subset deleted=w1127:string[])  [unwired: 1 out]
          }
        }
        n439 = Unbundle By Name(w1085) -> ("MES bool"=w1089:refnum<vi>)
        n440 = call "HD_Config.vi"("Step"=enum16{"Initial", "Write", "Read"}."Read") -> ("HD Config out"=w1088:T11)  [unwired: 9 in, 1 out]
        n441 = property class="Bool (严格)"(reference=w1089) -> ("Value"=w1091:bool)  [unwired: 1 in, 2 out]
        n442 = Unbundle By Name(w1088) -> ("Fail_resume_mode"=w1090:bool)
        n443 = call <vilib>:"Space Constant.vi"() -> ("String"=w1115:string)
        n444 = Not(x=w1091) -> (.not. x?=w1092:bool)
        n445 = Concatenate Strings(w1112, w1115, w1113) -> (w1114:string)
        n446 = Or(x=w1090, y=w1092) -> (x .or. y?=w1093:bool)
        n447 = Unbundle By Name(w1100) -> ("Initialisation.DDM_Parameter_status"=w1108:bool[], "Initialisation.Get_Tester_Parameter_status"=w1107:bool[])
        n448 = Index Array(array=w1076) -> (element #1=w1082:string, element #2=w1081:string, element #3=w1080:string)  [unwired: 3 in]
        n449 = Index Array(array=w1075) -> (element #1=w1077:string, element #2=w1078:string, element #3=w1079:string)  [unwired: 3 in]
        n450 = Bundle By Name(cluster=w1096, "daemon reference"=w1095, "Initialisation.Calculated Parameter - DDM Pressure Corrected"=w1082, "Initialisation.Calculated Parameter - DDM Real Power"=w1081, "Initialisation.Calculated Parameter - Delta V"=w1080, "Initialisation_Status.Calculated Parameter - DDM Pressure Corrected"=w1077, "Initialisation_Status.Calculated Parameter - DDM Real Power"=w1078, "Initialisation_Status.Calculated Parameter - Delta V"=w1079) -> (w1094:T1)
        n451 = Build Array (concatenate)(w1108, w1107, w1097) -> (w1106:bool[])
        n452 = Bundle By Name(cluster=w1100, "Initialisation.Cal_Tester_Parameter"=w1101, "Initialisation.Cal_Tester_Parameter_status"=w1097) -> (w1116:T3)
        n453 = And Array Elements(Boolean array=w1106) -> (logical AND=w1083:bool)
        n454 = Select(t=TRUE, s=w1093, f=w1083) -> (s? t:f=w1084:bool)
        n455 = call "LogStatus.vi"("error in (no error)"=w1120, "last message"=w1118, "message"=w1114) -> ("error  out"=w1119:errorcluster)  [unwired: 8 in]
        n456 = Select(t="Calibration_BEMF", s=w1084, f="Finalization_NG_unit") -> (s? t:f=w1102:string)
      }
      frame "Reflashing" {
        w1175 = "UIdisplay" ("Process (\"\" - local)")
        n457 = Unbundle By Name(w1160) -> ("Table"=w1174:string[][])
        n458 = call "Select_Table_Vaule Enable_Disable.vi"("Action"=w1172, "Table"=w1174) -> ("Enable"=w1166:bool)  [unwired: 8 in, 1 out]
        n459 = case shown="True" w1166 {
          tunnel: w1189 -> [w1192 w1205]
          tunnel: w1188 -> [_ w1204]
          tunnel: w1172 -> [w1191 w1203]
          tunnel: [w1192 w1201] -> w1187
          tunnel: w1186 -> [w1194 w1200]
          tunnel: [w1194 w1199] -> w1185
          tunnel: [w1193 w1197] -> w1184
          tunnel: [w1191 w1198] -> w1169
          tunnel: w1173 -> [w1193 w1197]
          tunnel: [w1190 w1195] -> w1161
          tunnel: w1160 -> [w1190 w1196]
          frame False {
          }
          frame True {
            n460 = call "LogStatus.vi"("error in (no error)"=w1205, "last message"=w1204, "message"=w1203) -> ("error  out"=w1202:errorcluster)  [unwired: 8 in]
            n461 = call "1.0.2_UUT_Reflashing.vi"("error in (no error)"=w1202, "Data in"=w1196, "Message Queue out"=w1200) -> ("error out"=w1201:errorcluster, "Flow"=w1198:string, "Data out"=w1195:T1, "Message Queue Out"=w1199:T4)  [unwired: 5 in]
          }
        }
        n462 = Select(t="Enable" ("元素"), s=w1166, f="Disable" ("元素")) -> (s? t:f=w1163:string)
        n463 = Flush Queue(queue=w1185) -> (queue out=w1162:T4)  [unwired: 1 in, 2 out]
        n464 = call "Select_Table_Vaule.vi"("Vaule"=w1163, "Action"=w1172, "Table"=w1174) -> ("Result"=w1182:bool, "vaule"=w1181:string[])  [unwired: 7 in]
        n465 = Append True/False String(1:w1182, 2:"FAIL" ("真字符串"), 3:"PASS" ("真字符串")) -> (0:w1180:string)  [unwired: 1 in]
        n466 = Build Array (concatenate)(w1181, w1163, w1180) -> (w1178:string[])
        n467 = Flatten To XML(anything=w1178) -> (xml string=w1179:string)
        n468 = call "AMC Send Local Message.vi"("Process (\"\" - local)"=w1175, "Message Value"=w1179, "Message Name"=w1175) -> ()  [unwired: 7 in, 2 out]
        n469 = Equal?(x=w1169, y="Disconnect_UUT") -> (x = y?=w1171:bool)
        n470 = Equal?(x=w1169, y="Error" ("Message Name")) -> (x = y?=w1167:bool)
        n471 = Or(x=w1171, y=w1167) -> (x .or. y?=w1168:bool)
      }
    }
    n472 = call "Stop.vi"("Step"=enum16{"Initial", "Write", "Read"}."Read") -> ("Stop Out"=w23:bool)  [unwired: 9 in, 1 out]
    n473 = call "Exit.vi"("Step"=enum16{"Initial", "Write", "Read"}."Read" ("step")) -> ("Exit Out"=w22:bool)  [unwired: 9 in, 1 out]
    n474 = call "6-AlarmStatus.vi"("Step"=enum16{"Initial", "Write", "Read"}."Read") -> ("AlarmValue Out"=w17:bool[])  [unwired: 9 in, 1 out]
    n475 = Or Array Elements(Boolean array=w17) -> (logical OR=w16:bool)
    n476 = call "AMC Run Step.vi"("Message Queue In"=w42, "Message Name"=w31, "Message Value"=w29, "error in (no error)"=w37, "Mli/Sig"=FALSE) -> ("Message Queue Out"=w41:T4, "error out"=w36:errorcluster)  [unwired: 13 in]
    n477 = Compound Arithmetic op=OR(w25, w23, w22, w16) -> (w24:bool)
  }
  "Message Queue Out" <- w6
  "error out" <- w5
  "Data" <- w9
  "Flow" <- w8
  "Data out" <- w2
